vi "2D_Plotter_MATLAB.vi"(1 "Job Directory":path) -> (2 "Saved Automatically?":bool, 3 "Error String":string, 4 "Plot data file":path)   [LabVIEW 2022 SP3]
uses:
  Controls/Global_mode.ctl
  Data plotting/MATLAB/MATLAB_Mode.ctl
  <vilib>/Analysis/baseanly.llb/Mean (DBL).vi
  <vilib>/Utility/error.llb/Trim Whitespace One-Sided.vi
  Results_plotter_Global.vi
  Globals/Constants_global.vi
  Data plotting/subVIs/Plot_Values_Global.vi
  <vilib>/Analysis/NI_AALBase.lvlib
panel:
  out "Show all Axis":bool
  out "Output format":string
  out "mSingleColorbar Actual":bool=TRUE
  out "Data Filenames":path[](array[path])
  out "Ord strngs":string[](array[string])
  out "Data Dir":string[](array[string])
  out "Output file":path
  out "Duplicate Plot":bool
  out "Source locations":string[](array[string])
  out "Selectors":i32[](array[numeric])
  out "Wind Directions":dbl[](array[numeric])
  out "Max dimension per figure":dbl[](array[numeric])
  out "Max Min array":dbl[][][](array[numeric])
  out "stl Limits":sgl[][](array[numeric])
  out "All Z":dbl[](array[numeric])
  out "All Y":dbl[](array[numeric])
  out "All X":dbl[](array[numeric])
  out "C limits":dbl[][](array[numeric])
  out "Plot Titles":string[](array[string])
  out "Number of Figures":i32
  out "Plot Y Axis":i32[](array[numeric])
  out "Plot X Axis":i32[](array[numeric])
  out "Limits Array":dbl[][][](array[numeric])
  out "Constant Axis":i32[](array[numeric])
  out "Plot":i32[](array[numeric])
  out "X Labels":bool[](array[boolean])
  out "Y labels":bool[](array[boolean])
  in  "Tab Control":T1(tab)
  in  "Show Save Option?":bool
  in  "Font Size":string="10"
  in  "MainTitleFontSize":string="12"
  in  "Height":string="0.02"
  in  "Width":string="0.2"
  in  "BottomEdge":string="0.05"
  in  "LeftEdge":string="0.4"
  in  "Flip vertical and Horizontal axes":bool
  in  "Auto":bool=TRUE
  in  "Number of Contours":i8=20 min=2 max=100
  in  "Interactive Window":bool
  in  "Show Source":bool
  in  "Source Size":string="300"
  in  "Source Color":string="r"
  in  "Source Z Location":u16(ring) items=["None", "Yaw (deg)", "Pitch (deg)", "P0 (Pa)", "P1 (Pa)", "P2 (Pa)", "P3 (Pa)", "P4 (Pa)", "P5 (Pa)", "P6 (Pa)", "Pstat (Pa)", "density for calculations", "P_ref (Pa)", "ngrid desired_resolution Polynomial_fitting", "OutputFile Decimal_Places", "Uref (m/s)", "density (kg/m^3)", "User Comments", "P_atmos (mbar)", "T_external (deg C)", "T_board (deg C)", "Humidity (%)", "ax (g)", "ay (g)", "az (g)", "wx (deg / s)", "wy (deg / s)", "wz (deg / s)", "Reference Temperature Used for Corrections", "Atmos Pressure Used for Corrections", "Raw Data Filename", "Multi Run Start Time", "P0/Pref", "P1/Pref", "P2/Pref", "P3/Pref", "P4/Pref", "P5/Pref", "P6/Pref", "P0 / P0", "P1 / P0", "P2 / P0", "P3 / P0", "P4 / P0", "P5 / P0", "P6 / P0", "File", "Current Filepath", "Template File Used", "Seconds since 1st Jan", "Mano (P0) Variance p0^2", "Mano (P1) Variance p1^2", "Mano (P2) Variance p2^2", "Mano (P3) Variance p3^2", "Mano (P4) Variance p4^2", "Mano (P5) Variance p5^2", "Mano (P6) Variance p6^2", "Date", "Mano (1P0) 1P0 Zero Offset", "Mano (1P1) 1P1 Zero Offset", "Mano (1P2) 1P2 Zero Offset", "Mano (1P3) 1P3 Zero Offset", "Mano (1P4) 1P4 Zero Offset", "Mano (1P5) 1P5 Zero Offset", "Mano (1P6) 1P6 Zero Offset", "Speed Calib Tweak", "Speed Dem Voltage", "Run Description", "Multi Run Row Number", "P0 (Pa) Std Error", "P1 (Pa) Std Error", "P2 (Pa) Std Error", "P3 (Pa) Std Error", "P4 (Pa) Std Error", "P5 (Pa) Std Error", "P6 (Pa) Std Error", "P0/Pref Std Error", "P1/Pref Std Error", "P2/Pref Std Error", "P3/Pref Std Error", "P4/Pref Std Error", "P5/Pref Std Error", "P6/Pref Std Error", "Flow Measurement Time"]
  in  "Source Y Location":u16(ring) items=["None", "Yaw (deg)", "Pitch (deg)", "P0 (Pa)", "P1 (Pa)", "P2 (Pa)", "P3 (Pa)", "P4 (Pa)", "P5 (Pa)", "P6 (Pa)", "Pstat (Pa)", "density for calculations", "P_ref (Pa)", "ngrid desired_resolution Polynomial_fitting", "OutputFile Decimal_Places", "Uref (m/s)", "density (kg/m^3)", "User Comments", "P_atmos (mbar)", "T_external (deg C)", "T_board (deg C)", "Humidity (%)", "ax (g)", "ay (g)", "az (g)", "wx (deg / s)", "wy (deg / s)", "wz (deg / s)", "Reference Temperature Used for Corrections", "Atmos Pressure Used for Corrections", "Raw Data Filename", "Multi Run Start Time", "P0/Pref", "P1/Pref", "P2/Pref", "P3/Pref", "P4/Pref", "P5/Pref", "P6/Pref", "P0 / P0", "P1 / P0", "P2 / P0", "P3 / P0", "P4 / P0", "P5 / P0", "P6 / P0", "File", "Current Filepath", "Template File Used", "Seconds since 1st Jan", "Mano (P0) Variance p0^2", "Mano (P1) Variance p1^2", "Mano (P2) Variance p2^2", "Mano (P3) Variance p3^2", "Mano (P4) Variance p4^2", "Mano (P5) Variance p5^2", "Mano (P6) Variance p6^2", "Date", "Mano (1P0) 1P0 Zero Offset", "Mano (1P1) 1P1 Zero Offset", "Mano (1P2) 1P2 Zero Offset", "Mano (1P3) 1P3 Zero Offset", "Mano (1P4) 1P4 Zero Offset", "Mano (1P5) 1P5 Zero Offset", "Mano (1P6) 1P6 Zero Offset", "Speed Calib Tweak", "Speed Dem Voltage", "Run Description", "Multi Run Row Number", "P0 (Pa) Std Error", "P1 (Pa) Std Error", "P2 (Pa) Std Error", "P3 (Pa) Std Error", "P4 (Pa) Std Error", "P5 (Pa) Std Error", "P6 (Pa) Std Error", "P0/Pref Std Error", "P1/Pref Std Error", "P2/Pref Std Error", "P3/Pref Std Error", "P4/Pref Std Error", "P5/Pref Std Error", "P6/Pref Std Error", "Flow Measurement Time"]
  in  "Source X Location":u16(ring) items=["None", "Yaw (deg)", "Pitch (deg)", "P0 (Pa)", "P1 (Pa)", "P2 (Pa)", "P3 (Pa)", "P4 (Pa)", "P5 (Pa)", "P6 (Pa)", "Pstat (Pa)", "density for calculations", "P_ref (Pa)", "ngrid desired_resolution Polynomial_fitting", "OutputFile Decimal_Places", "Uref (m/s)", "density (kg/m^3)", "User Comments", "P_atmos (mbar)", "T_external (deg C)", "T_board (deg C)", "Humidity (%)", "ax (g)", "ay (g)", "az (g)", "wx (deg / s)", "wy (deg / s)", "wz (deg / s)", "Reference Temperature Used for Corrections", "Atmos Pressure Used for Corrections", "Raw Data Filename", "Multi Run Start Time", "P0/Pref", "P1/Pref", "P2/Pref", "P3/Pref", "P4/Pref", "P5/Pref", "P6/Pref", "P0 / P0", "P1 / P0", "P2 / P0", "P3 / P0", "P4 / P0", "P5 / P0", "P6 / P0", "File", "Current Filepath", "Template File Used", "Seconds since 1st Jan", "Mano (P0) Variance p0^2", "Mano (P1) Variance p1^2", "Mano (P2) Variance p2^2", "Mano (P3) Variance p3^2", "Mano (P4) Variance p4^2", "Mano (P5) Variance p5^2", "Mano (P6) Variance p6^2", "Date", "Mano (1P0) 1P0 Zero Offset", "Mano (1P1) 1P1 Zero Offset", "Mano (1P2) 1P2 Zero Offset", "Mano (1P3) 1P3 Zero Offset", "Mano (1P4) 1P4 Zero Offset", "Mano (1P5) 1P5 Zero Offset", "Mano (1P6) 1P6 Zero Offset", "Speed Calib Tweak", "Speed Dem Voltage", "Run Description", "Multi Run Row Number", "P0 (Pa) Std Error", "P1 (Pa) Std Error", "P2 (Pa) Std Error", "P3 (Pa) Std Error", "P4 (Pa) Std Error", "P5 (Pa) Std Error", "P6 (Pa) Std Error", "P0/Pref Std Error", "P1/Pref Std Error", "P2/Pref Std Error", "P3/Pref Std Error", "P4/Pref Std Error", "P5/Pref Std Error", "P6/Pref Std Error", "Flow Measurement Time"]
  in  "Rotate Model?":bool
  in  "Vectors":bool
  in  "Streamlines":bool
  in  "W Vector":u16(ring) items=["None", "Yaw (deg)", "Pitch (deg)", "P0 (Pa)", "P1 (Pa)", "P2 (Pa)", "P3 (Pa)", "P4 (Pa)", "P5 (Pa)", "P6 (Pa)", "Pstat (Pa)", "density for calculations", "P_ref (Pa)", "ngrid desired_resolution Polynomial_fitting", "OutputFile Decimal_Places", "Uref (m/s)", "density (kg/m^3)", "User Comments", "P_atmos (mbar)", "T_external (deg C)", "T_board (deg C)", "Humidity (%)", "ax (g)", "ay (g)", "az (g)", "wx (deg / s)", "wy (deg / s)", "wz (deg / s)", "Reference Temperature Used for Corrections", "Atmos Pressure Used for Corrections", "Raw Data Filename", "Multi Run Start Time", "P0/Pref", "P1/Pref", "P2/Pref", "P3/Pref", "P4/Pref", "P5/Pref", "P6/Pref", "P0 / P0", "P1 / P0", "P2 / P0", "P3 / P0", "P4 / P0", "P5 / P0", "P6 / P0", "File", "Current Filepath", "Template File Used", "Seconds since 1st Jan", "Mano (P0) Variance p0^2", "Mano (P1) Variance p1^2", "Mano (P2) Variance p2^2", "Mano (P3) Variance p3^2", "Mano (P4) Variance p4^2", "Mano (P5) Variance p5^2", "Mano (P6) Variance p6^2", "Date", "Mano (1P0) 1P0 Zero Offset", "Mano (1P1) 1P1 Zero Offset", "Mano (1P2) 1P2 Zero Offset", "Mano (1P3) 1P3 Zero Offset", "Mano (1P4) 1P4 Zero Offset", "Mano (1P5) 1P5 Zero Offset", "Mano (1P6) 1P6 Zero Offset", "Speed Calib Tweak", "Speed Dem Voltage", "Run Description", "Multi Run Row Number", "P0 (Pa) Std Error", "P1 (Pa) Std Error", "P2 (Pa) Std Error", "P3 (Pa) Std Error", "P4 (Pa) Std Error", "P5 (Pa) Std Error", "P6 (Pa) Std Error", "P0/Pref Std Error", "P1/Pref Std Error", "P2/Pref Std Error", "P3/Pref Std Error", "P4/Pref Std Error", "P5/Pref Std Error", "P6/Pref Std Error", "Flow Measurement Time"]
  in  "U Vector":u16(ring) items=["None", "Yaw (deg)", "Pitch (deg)", "P0 (Pa)", "P1 (Pa)", "P2 (Pa)", "P3 (Pa)", "P4 (Pa)", "P5 (Pa)", "P6 (Pa)", "Pstat (Pa)", "density for calculations", "P_ref (Pa)", "ngrid desired_resolution Polynomial_fitting", "OutputFile Decimal_Places", "Uref (m/s)", "density (kg/m^3)", "User Comments", "P_atmos (mbar)", "T_external (deg C)", "T_board (deg C)", "Humidity (%)", "ax (g)", "ay (g)", "az (g)", "wx (deg / s)", "wy (deg / s)", "wz (deg / s)", "Reference Temperature Used for Corrections", "Atmos Pressure Used for Corrections", "Raw Data Filename", "Multi Run Start Time", "P0/Pref", "P1/Pref", "P2/Pref", "P3/Pref", "P4/Pref", "P5/Pref", "P6/Pref", "P0 / P0", "P1 / P0", "P2 / P0", "P3 / P0", "P4 / P0", "P5 / P0", "P6 / P0", "File", "Current Filepath", "Template File Used", "Seconds since 1st Jan", "Mano (P0) Variance p0^2", "Mano (P1) Variance p1^2", "Mano (P2) Variance p2^2", "Mano (P3) Variance p3^2", "Mano (P4) Variance p4^2", "Mano (P5) Variance p5^2", "Mano (P6) Variance p6^2", "Date", "Mano (1P0) 1P0 Zero Offset", "Mano (1P1) 1P1 Zero Offset", "Mano (1P2) 1P2 Zero Offset", "Mano (1P3) 1P3 Zero Offset", "Mano (1P4) 1P4 Zero Offset", "Mano (1P5) 1P5 Zero Offset", "Mano (1P6) 1P6 Zero Offset", "Speed Calib Tweak", "Speed Dem Voltage", "Run Description", "Multi Run Row Number", "P0 (Pa) Std Error", "P1 (Pa) Std Error", "P2 (Pa) Std Error", "P3 (Pa) Std Error", "P4 (Pa) Std Error", "P5 (Pa) Std Error", "P6 (Pa) Std Error", "P0/Pref Std Error", "P1/Pref Std Error", "P2/Pref Std Error", "P3/Pref Std Error", "P4/Pref Std Error", "P5/Pref Std Error", "P6/Pref Std Error", "Flow Measurement Time"]
  in  "V Vector":u16(ring) items=["None", "Yaw (deg)", "Pitch (deg)", "P0 (Pa)", "P1 (Pa)", "P2 (Pa)", "P3 (Pa)", "P4 (Pa)", "P5 (Pa)", "P6 (Pa)", "Pstat (Pa)", "density for calculations", "P_ref (Pa)", "ngrid desired_resolution Polynomial_fitting", "OutputFile Decimal_Places", "Uref (m/s)", "density (kg/m^3)", "User Comments", "P_atmos (mbar)", "T_external (deg C)", "T_board (deg C)", "Humidity (%)", "ax (g)", "ay (g)", "az (g)", "wx (deg / s)", "wy (deg / s)", "wz (deg / s)", "Reference Temperature Used for Corrections", "Atmos Pressure Used for Corrections", "Raw Data Filename", "Multi Run Start Time", "P0/Pref", "P1/Pref", "P2/Pref", "P3/Pref", "P4/Pref", "P5/Pref", "P6/Pref", "P0 / P0", "P1 / P0", "P2 / P0", "P3 / P0", "P4 / P0", "P5 / P0", "P6 / P0", "File", "Current Filepath", "Template File Used", "Seconds since 1st Jan", "Mano (P0) Variance p0^2", "Mano (P1) Variance p1^2", "Mano (P2) Variance p2^2", "Mano (P3) Variance p3^2", "Mano (P4) Variance p4^2", "Mano (P5) Variance p5^2", "Mano (P6) Variance p6^2", "Date", "Mano (1P0) 1P0 Zero Offset", "Mano (1P1) 1P1 Zero Offset", "Mano (1P2) 1P2 Zero Offset", "Mano (1P3) 1P3 Zero Offset", "Mano (1P4) 1P4 Zero Offset", "Mano (1P5) 1P5 Zero Offset", "Mano (1P6) 1P6 Zero Offset", "Speed Calib Tweak", "Speed Dem Voltage", "Run Description", "Multi Run Row Number", "P0 (Pa) Std Error", "P1 (Pa) Std Error", "P2 (Pa) Std Error", "P3 (Pa) Std Error", "P4 (Pa) Std Error", "P5 (Pa) Std Error", "P6 (Pa) Std Error", "P0/Pref Std Error", "P1/Pref Std Error", "P2/Pref Std Error", "P3/Pref Std Error", "P4/Pref Std Error", "P5/Pref Std Error", "P6/Pref Std Error", "Flow Measurement Time"]
  in  "Stl File":u16(ring) items=["", "Case1.stl", "Case2.stl", "Case2a.stl", "Case2b.stl", "Case2c.stl", "Case3.stl", "MagicBuildingswithRoofs.stl", "StreetCanyonGeometry.stl", "Veg_Barrier_EmptyCanyon.stl", "Veg_Barrier_tree_nospacing.stl", "Veg_Barrier_tree_spacing.stl"]
  out "Y Limit":string
  out "X Limit":string
  in  "Concentration?":bool
  in  "Range Auto":bool=TRUE
  in  "Same Location limits for all plots":bool=TRUE
  in  "Swop Series and Plots":bool
  in  "mSingleColorbar":bool=TRUE
  in  "Y Limits Auto":bool=TRUE
  in  "X Limits Auto":bool=TRUE
  in  "cContourAct":bool=TRUE
  in  "Location X limits":string="-2000;2000"
  out "stl file":string
  in  "nRows":u8=3 min=1
  in  "nCols":u8=3 min=1
  in  "cScatterAct":bool=TRUE
  in  "cScatterPointSize":string="5"
  in  "Plotting":enum8{"Lin", "Log"}(ring)
  in  "fvectorRotation":string="0;0;0"
  in  "cdColorbarRange":string="0.01;100"
  in  "No Of decades":i32=3 min=1 max=10
  in  "Location Y limits":string="-2000;2000"
  in  "Open in Acrobat":bool=TRUE
  in  "Reduce Individual Plot Title Lengths if too long":bool=TRUE
  in  "Show Channels with range of Values?":bool
  in  "Page Title Pre Block":string
  in  "Page Title Post Block":string
  in  "Values to include in Page Title":i32[](listbox)
  out "Final Title":string
  in  "Math titles":bool=TRUE
  out "Plot Legends Auto":string[](array[string])
  out "No of Series supplied":i32
  out "AuditTrail":string[](array[string])
  out "Desired Legends":string[][](array[string])
  out "Table":string[][](table)
  # "Plot XY axes control"
  # "Color Bar"
  # "Overall Page Title"
  # "There are as many graphs as there are titles (from Selector 2)...."
  # "Plot Styles"
  # "Each graph contains plots from Selector 1..."
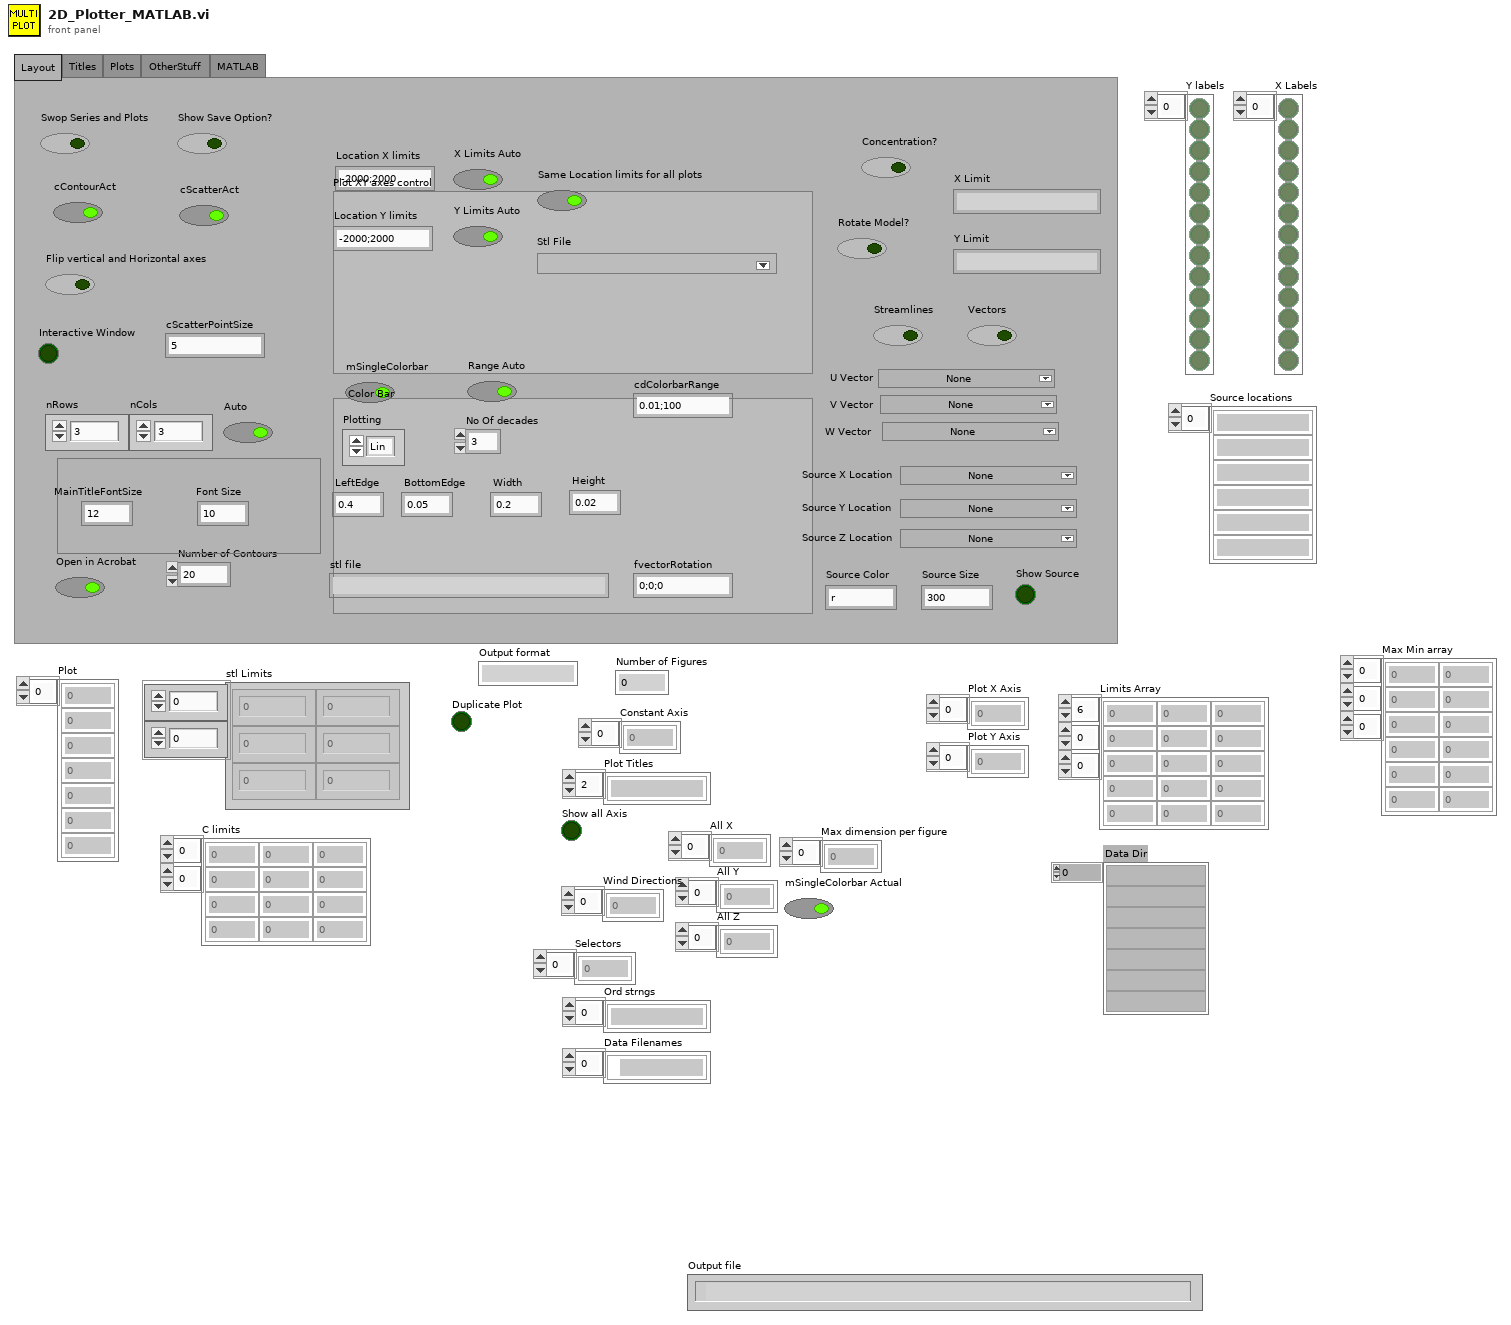
[diagram p1: front panel]
types:
  T1 = enum32{"Layout", "Titles", "Plots", "OtherStuff ", "MATLAB"}
  T2 = typedef "Global_mode.ctl" = enum16{"Read Global", "Load Global From File", "Write Global to File"}
  T3 = typedef "MATLAB_Mode.ctl" = enum16{"1D Plotter", "2D Plotter", "LP Plotter", "7HP UVW"}
  T4 = typedef "RFP_Plot_Metadata.ctl" = cluster{"Row Number":i32[], "Error Bars":T5, "X Label":string, "Y Label":string, "Blanks NaNs":i32[]}
  T5 = typedef "Error_bars_index.ctl" = cluster{"Upper":i32, "Lower":i32, "St Error":i32}
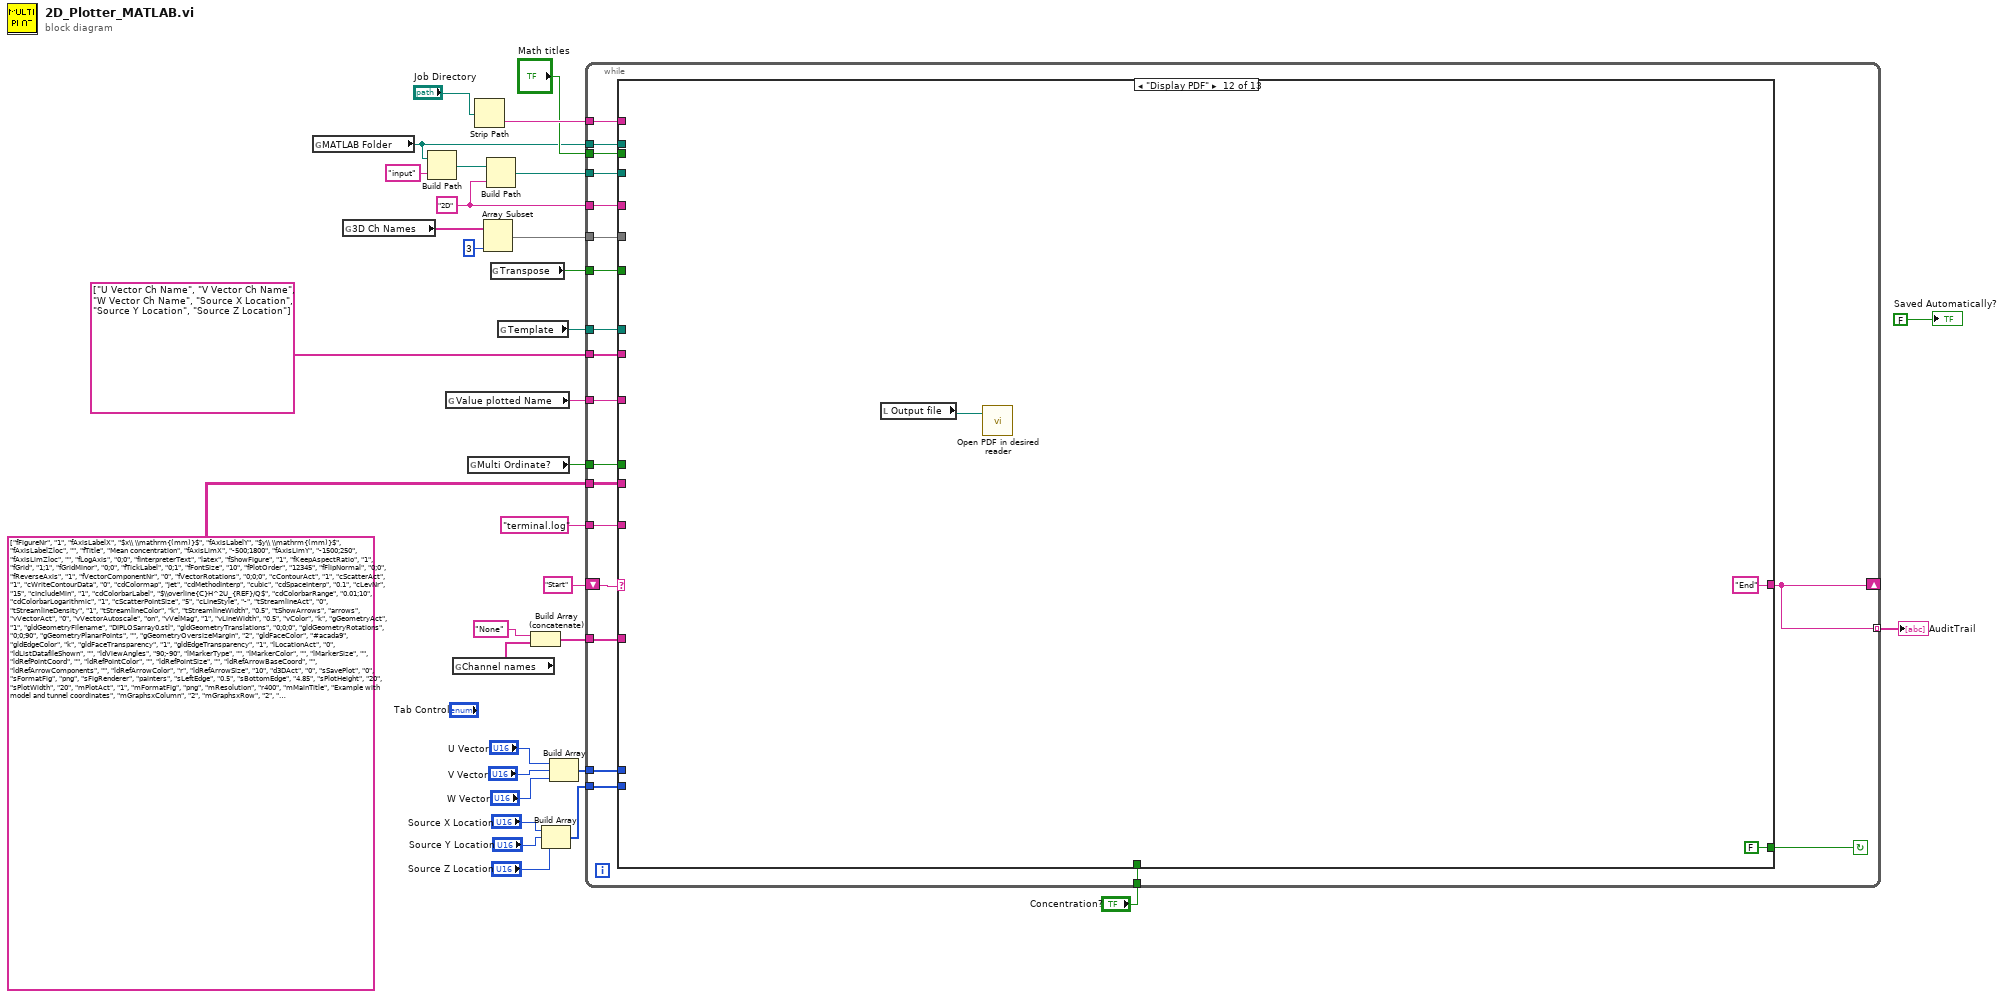
[diagram p0: block diagram]
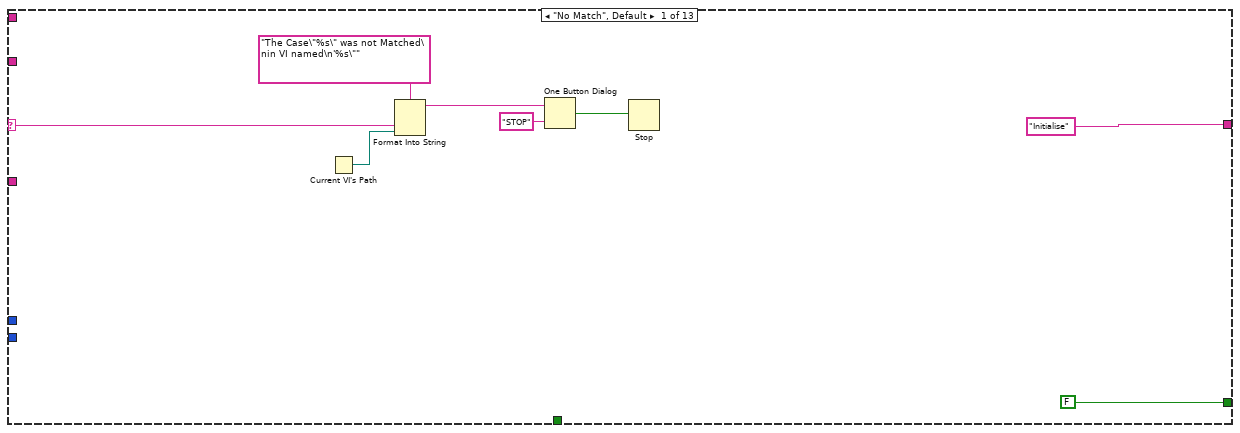
[diagram p2: hidden frame]
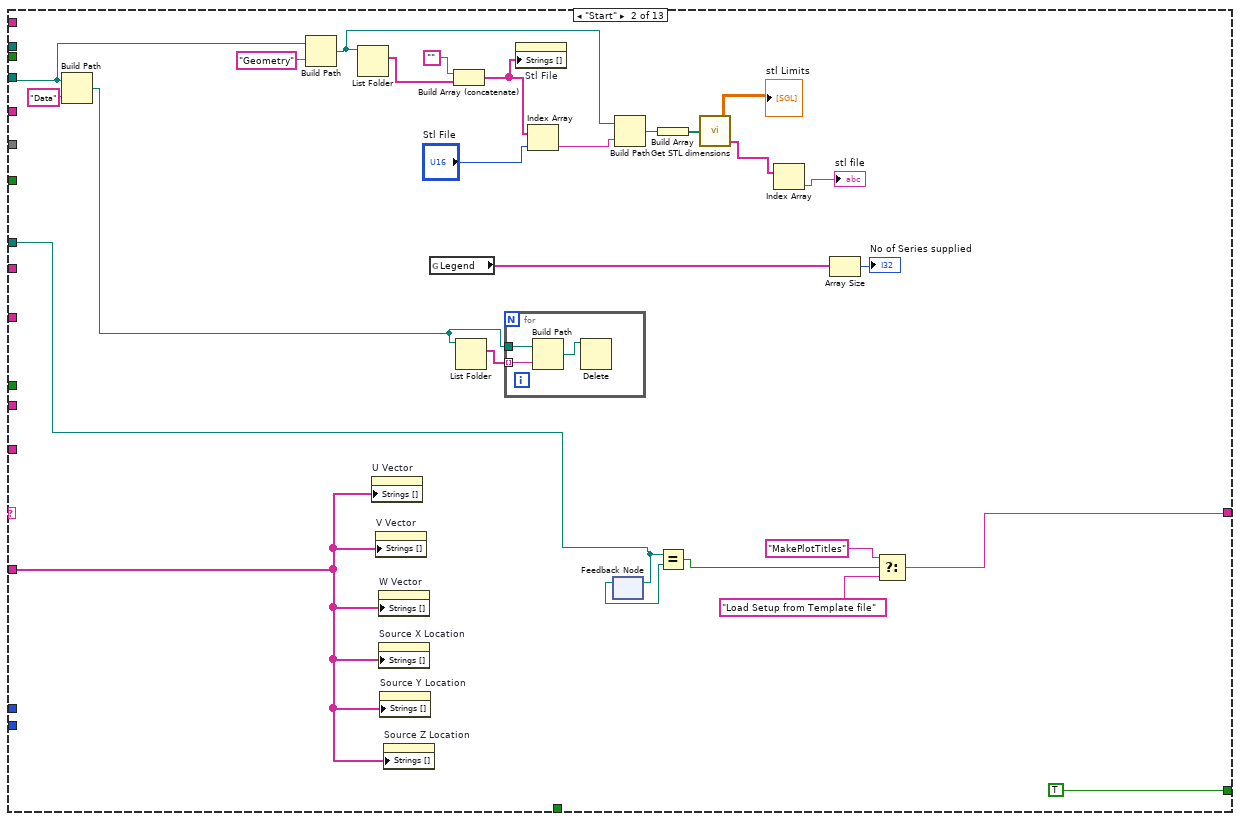
[diagram p3: hidden frame]
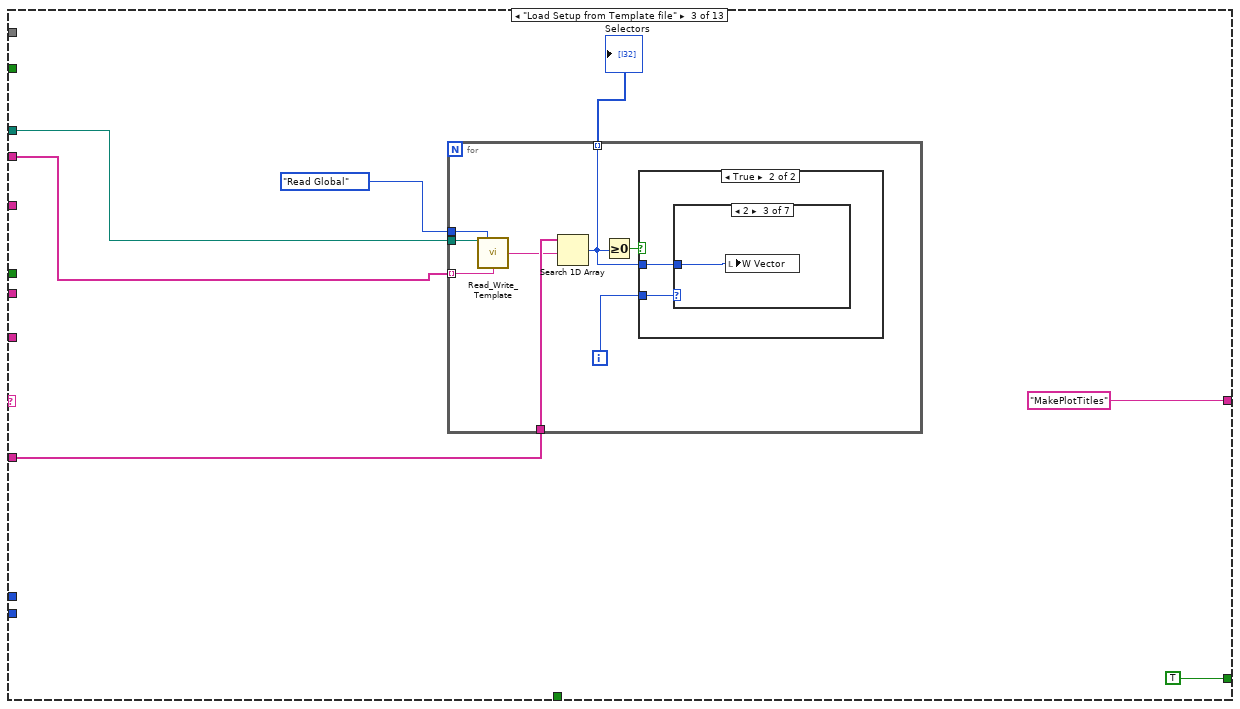
[diagram p4: hidden frame]
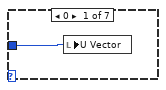
[diagram p6: hidden frame]
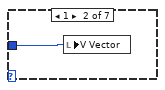
[diagram p7: hidden frame]
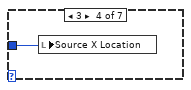
[diagram p8: hidden frame]
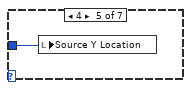
[diagram p9: hidden frame]
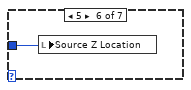
[diagram p10: hidden frame]
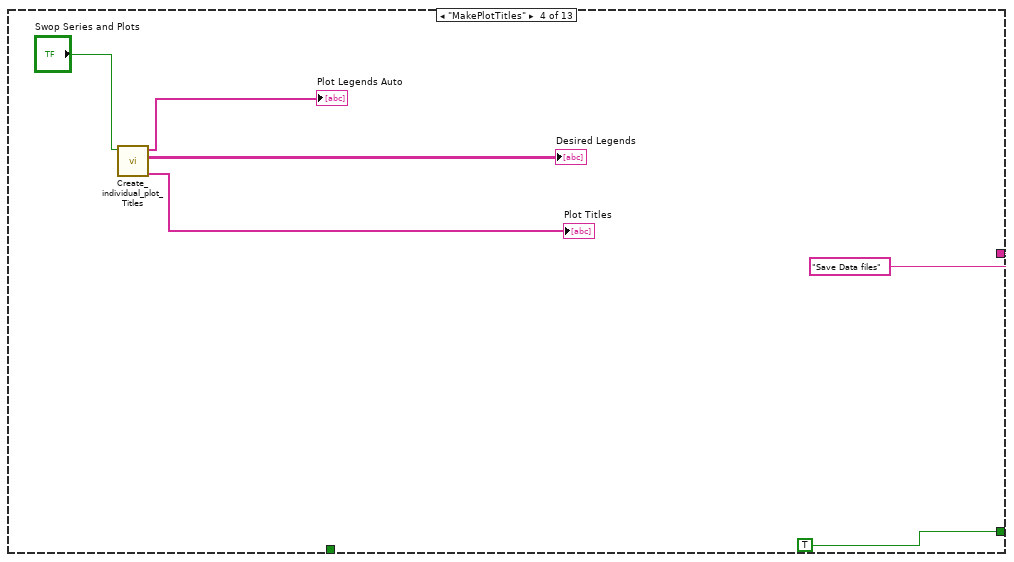
[diagram p12: hidden frame]
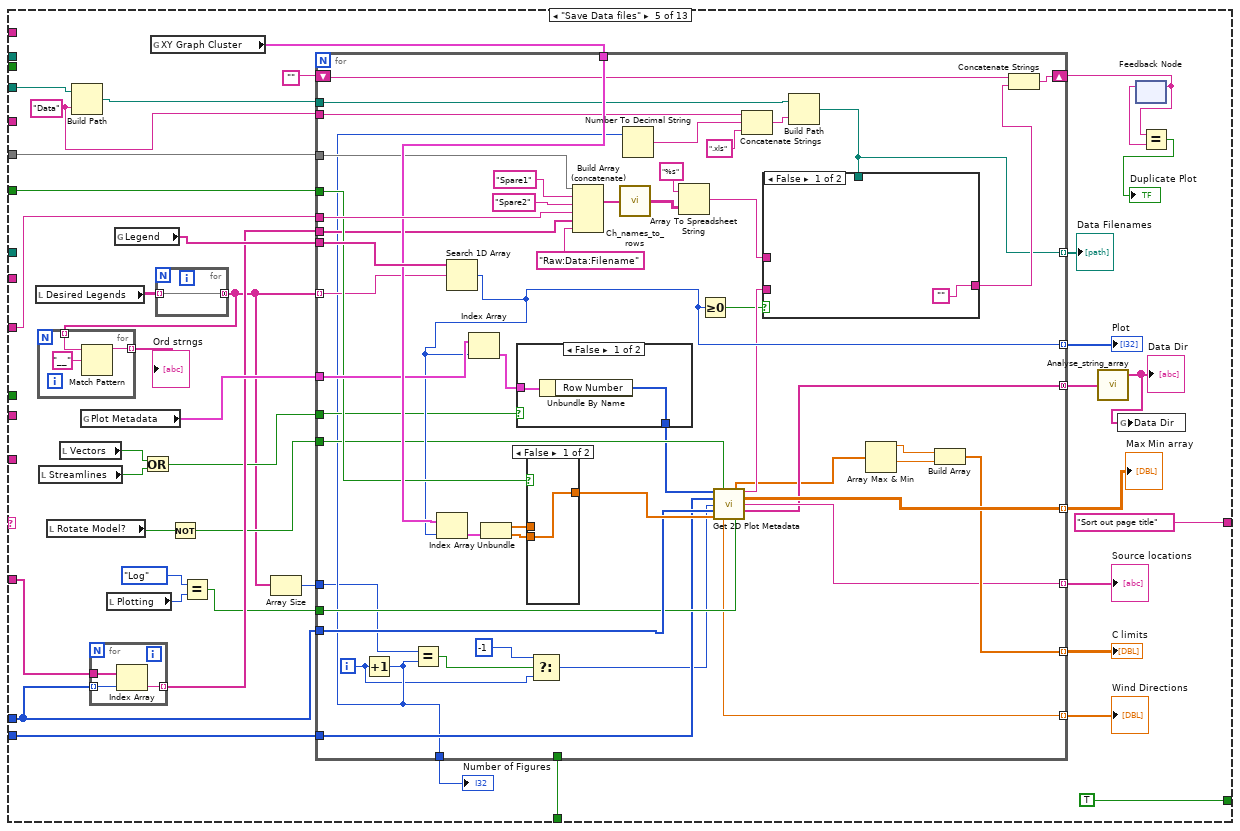
[diagram p13: hidden frame]
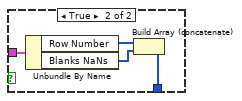
[diagram p14: hidden frame]
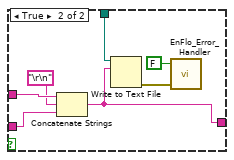
[diagram p16: hidden frame]
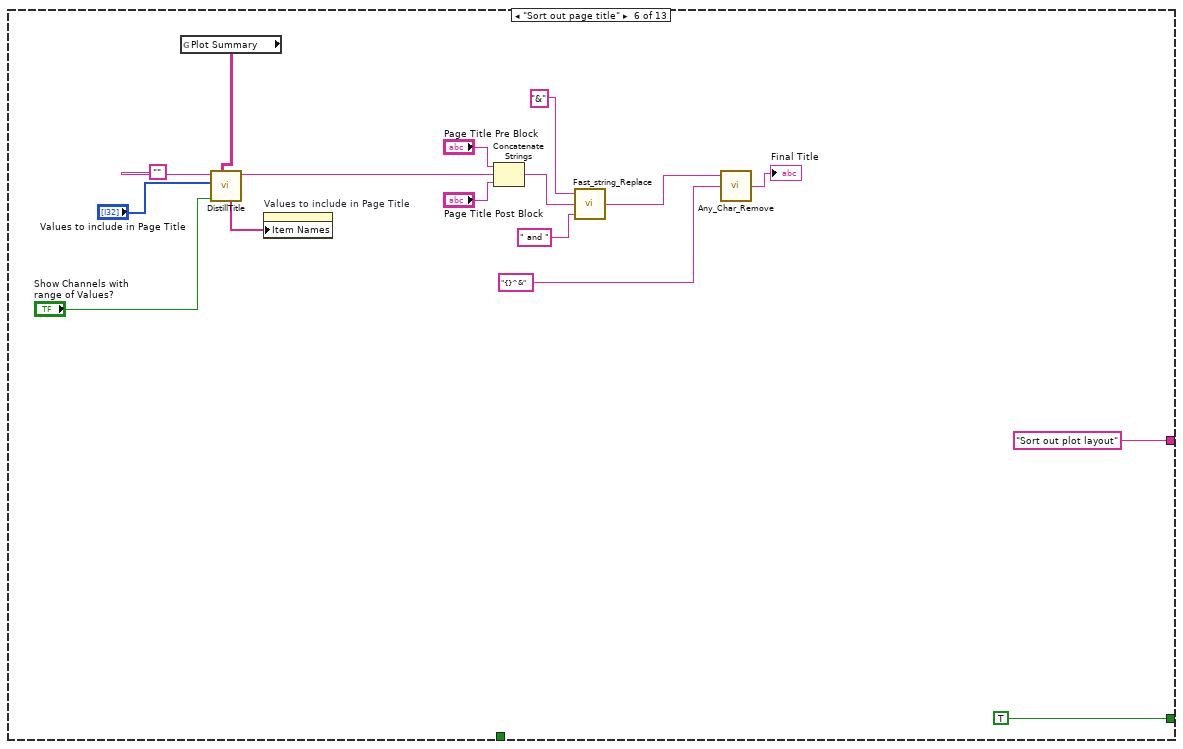
[diagram p17: hidden frame]
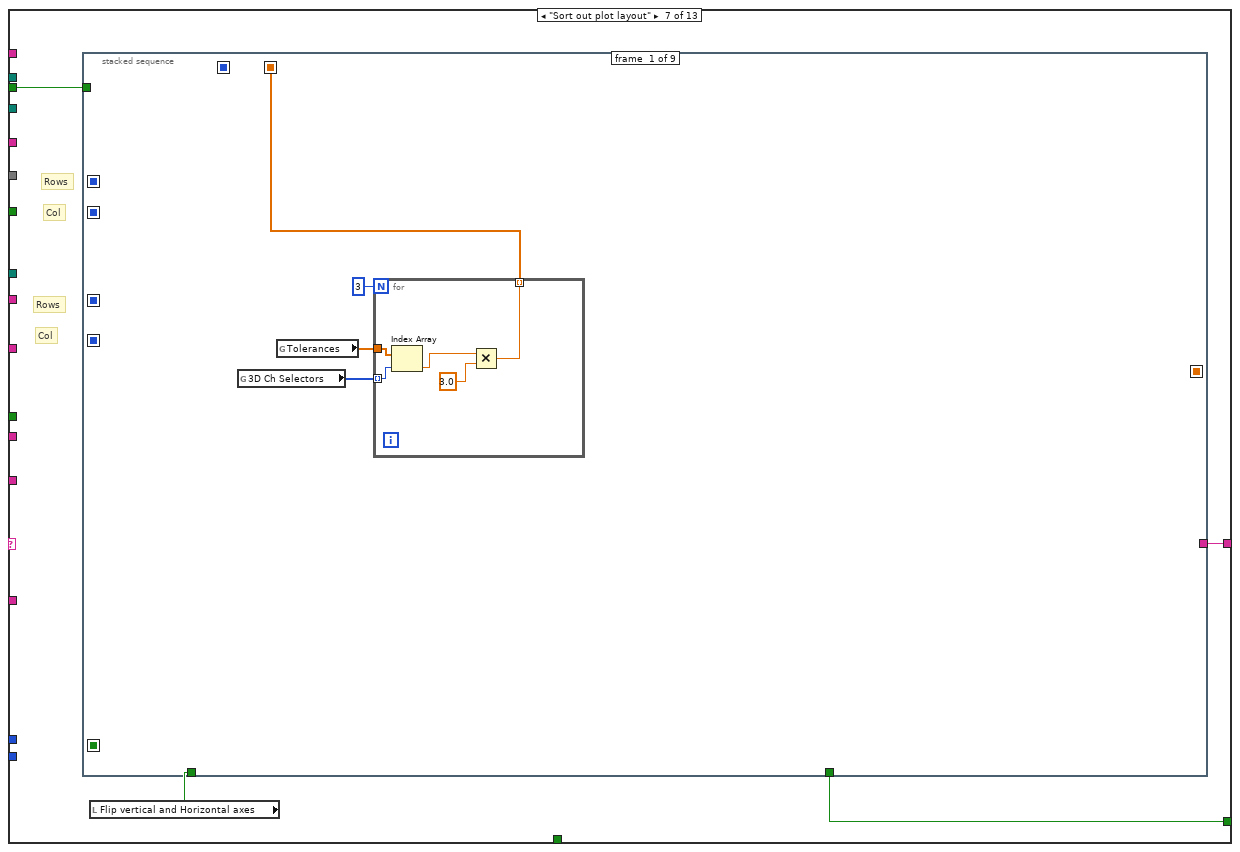
[diagram p18: hidden frame]
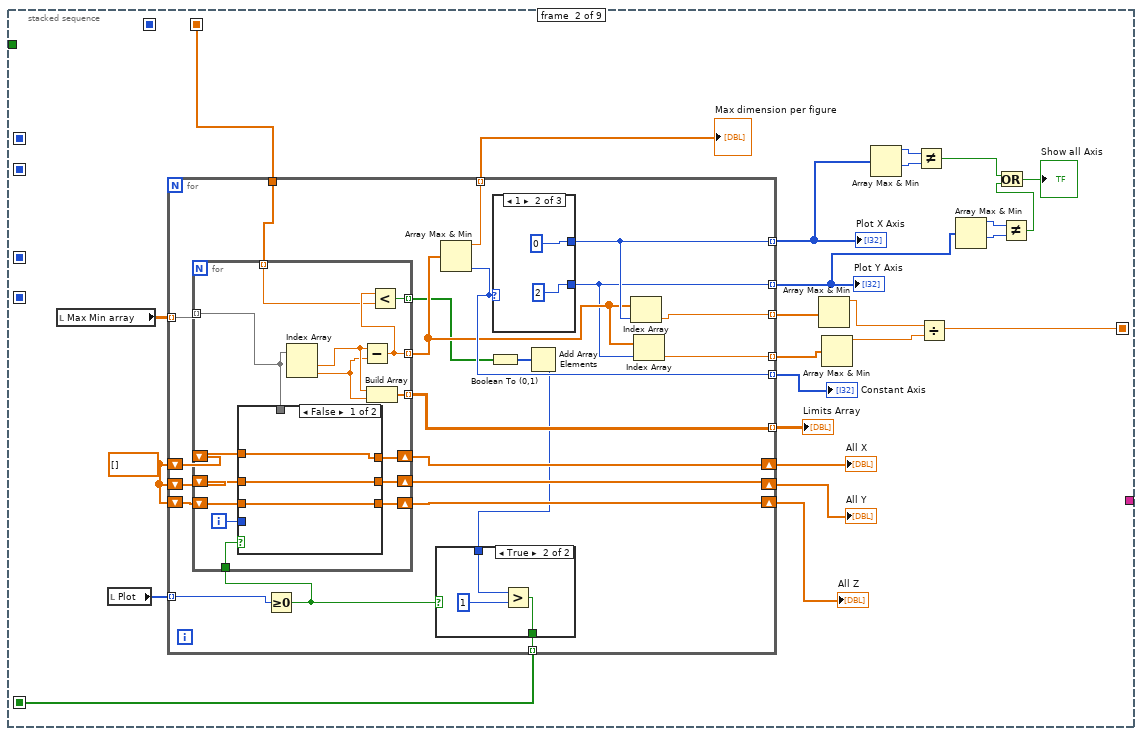
[diagram p19: hidden frame]
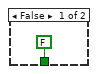
[diagram p20: hidden frame]
diagram:
  w1 = "2D" ("name or relative path")
  n1 = global read "Constants_global.vi" "MATLAB Folder"() -> (w2:path)
  n2 = global read "Results_plotter_Global.vi" "3D Ch Names"() -> (w13:string[])
  n3 = Build Path(base path=w2, name or relative path="input") -> (appended path=w25:path)
  n4 = global read "Results_plotter_Global.vi" "Value plotted Name"() -> (w32:string)
  n5 = global read "Results_plotter_Global.vi" "Channel names"() -> (w21:string[])
  n6 = global read "Results_plotter_Global.vi" "Multi Ordinate?"() -> (w28:bool)
  n7 = Strip Path(path="Job Directory") -> (name=w4:string)  [unwired: 1 out]
  n8 = Array Subset(array=w13, length=3) -> (w12:string[])  [unwired: 1 in]
  n9 = Build Path(base path=w25, name or relative path=w1) -> (appended path=w24:path)
  n10 = global read "Results_plotter_Global.vi" "Transpose"() -> (w29:bool)
  n11 = global read "Results_plotter_Global.vi" "Template"() -> (w11:path)
  n12 = Build Array (concatenate)("None", w21) -> (w19:string[])
  n13 = Build Array("Source X Location", "Source Y Location", "Source Z Location") -> (w6:u16[])
  n14 = Build Array("U Vector", "V Vector", "W Vector") -> (w15:u16[])
  n15 = while {
    shift-left: "Start" -> [w52]
    shift-right: [w47] -> _
    tunnel: w32 -> [w51]
    tunnel: "terminal.log" -> [w50]
    tunnel: w29 -> [w49]
    tunnel: w28 -> [w48]
    tunnel: [w47] -> w27 mode=indexing
    tunnel: w24 -> [w46]
    tunnel: string[][] [["fFigureNr", "1"], ["fAxisLabelX", "$x\\ \\mathrm{(mm)}$"], ["fAxisLabelY", "$y\\ \\mathrm{(mm)}$"], ["fAxisLabelZloc", ""], ["fTitle", "Mean concentration"], ["fAxisLimX", "-500;1800"], ["fAxisLimY", "-1500;250"], ["fAxisLimZloc", ""], ["fLogAxis", "0;0"], ["fInterpreterText", "latex"], ["fShowFigure", "1"], ["fKeepAspectRatio", "1"], ["fGrid", "1;1"], ["fGridMinor", "0;0"], ["fTickLabel", "0;1"], ["fFontSize", "10"], ["fPlotOrder", "12345"], ["fFlipNormal", "0;0"], ["fReverseAxis", "1"], ["fVectorComponentNr", "0"], ["fVectorRotations", "0;0;0"], ["cContourAct", "1"], ["cScatterAct", "1"], ["cWriteContourData", "0"], ["cdColormap", "jet"], ["cdMethodInterp", "cubic"], ["cdSpaceInterp", "0.1"], ["cLevNr", "15"], ["cIncludeMin", "1"], ["cdColorbarLabel", "$\\overline{C}H^2U_{REF}/Q$"], ["cdColorbarRange", "0.01;10"], ["cdColorbarLogarithmic", "1"], ["cScatterPointSize", "5"], ["cLineStyle", "-"], ["tStreamlineAct", "0"], ["tStreamlineDensity", "1"], ["tStreamlineColor", "k"], ["tStreamlineWidth", "0.5"], ["tShowArrows", "arrows"], ["vVectorAct", "0"], ["vVectorAutoscale", "on"], ["vVelMag", "1"], ["vLineWidth", "0.5"], ["vColor", "k"], ["gGeometryAct", "1"], ["gldGeometryFilename", "DIPLOSarray0.stl"], ["gldGeometryTranslations", "0;0;0"], ["gldGeometryRotations", "0;0;90"], ["gGeometryPlanarPoints", ""], ["gGeometryOversizeMargin", "2"], ["gldFaceColor", "#acada9"], ["gldEdgeColor", "k"], ["gldFaceTransparency", "1"], ["gldEdgeTransparency", "1"], ["lLocationAct", "0"], ["ldListDatafileShown", ""], ["ldViewAngles", "90;-90"], ["lMarkerType", ""], ["lMarkerColor", ""], ["lMarkerSize", ""], ["ldRefPointCoord", ""], ["ldRefPointColor", ""], ["ldRefPointSize", ""], ["ldRefArrowBaseCoord", ""], ["ldRefArrowComponents", ""], ["ldRefArrowColor", "r"], ["ldRefArrowSize", "10"], ["d3DAct", "0"], ["sSavePlot", "0"], ["sFormatFig", "png"], ["sFigRenderer", "painters"], ["sLeftEdge", "0.5"], ["sBottomEdge", "4.85"], ["sPlotHeight", "20"], ["sPlotWidth", "20"], ["mPlotAct", "1"], ["mFormatFig", "png"], ["mResolution", "r400"], ["mMainTitle", "Example with model and tunnel coordinates"], ["mGraphsxColumn", "2"], ["mGraphsxRow", "2"], ["mLeftEdge", "1.8"], ["mRightEdge", "0.8"], ["mTopEdge", "1.5"], ["mBottomEdge", "1.5"], ["mSpaceX", "0.1"], ["mSpaceY", "0.5"], ["mPlotHeight", "21"], ["mPlotWidth", "29.7"], ["mMainTitleFontSize", "12"], ["mFontSize", "10"], ["mInterpreterText", "latex"], ["mFigRenderer", "opengl"], ["mSingleColorbar", "1"], ["mSingleColorbarOrientation", "Horizontal"], ["mSingleColorbarLocation", "0.4;0.05;0.2;0.02"], ["dStreamlineSlice", "2"], ["dStreamlineStartPoint1", "0;0;0.5"], ["dStreamlineStartPoint2", "0;1;0.5"], ["dContourTransparency", "1"]] ("appended array") -> [w45]
    tunnel: "Concentration?" -> [w44]
    tunnel: w19 -> [w43]
    tunnel: w15 -> [w42]
    tunnel: w12 -> [w41]
    tunnel: w11 -> [w40]
    tunnel: string[] ["U Vector Ch Name", "V Vector Ch Name", "W Vector Ch Name", "Source X Location", "Source Y Location", "Source Z Location"] -> [w39]
    tunnel: w6 -> [w38]
    tunnel: w4 -> [w37]
    tunnel: "Math titles" -> [w36]
    tunnel: w2 -> [w35]
    tunnel: w1 -> [w34]
    stop <- w53 continue-if-true
    n16 = case shown="\"Display PDF\"" w52 {
      selector: w52 -> [w54 _ _ _ _ _ _ _ _ _ _ _ _]
      tunnel: [FALSE TRUE TRUE ("Top Level") TRUE ("Top Level") TRUE ("Top Level") TRUE ("Top Level") w255 TRUE ("Top Level") TRUE ("Top Level") w1307 FALSE ("Top Level") FALSE ("Top Level") FALSE ("Top Level")] -> w53
      tunnel: ["Initialise" w68 "MakePlotTitles" "Save Data files" "Sort out page title" "Sort out plot layout" w253 "Save Input File" ("t") "Run MATLAB Code" ("t") w1300 "" "End" ("t") "End" ("t")] -> w47
      tunnel: w51 -> [_ _ _ _ w150 _ _ _ _ _ _ _ _]
      tunnel: w50 -> [_ _ _ _ _ _ _ _ _ _ _ _ _]
      tunnel: w49 -> [_ _ _ _ w160 _ _ _ _ _ _ _ _]
      tunnel: w48 -> [_ _ _ _ _ _ _ _ _ _ _ _ _]
      tunnel: w46 -> [_ w78 _ _ w154 _ _ w792 w1280 _ _ _ _]
      tunnel: w45 -> [_ _ _ _ _ _ _ w799 _ _ _ _ _]
      tunnel: w44 -> [_ _ _ _ w147 _ _ _ _ _ _ _ _]
      tunnel: w43 -> [_ w65 w94 _ w146 _ _ _ w1268 _ _ _ _]
      tunnel: w42 -> [_ _ _ _ w144 _ _ _ _ _ _ _ _]
      tunnel: w41 -> [_ _ _ _ w143 _ _ _ _ _ _ _ _]
      tunnel: w40 -> [_ w66 w95 _ _ _ _ _ w1270 _ _ _ _]
      tunnel: w39 -> [_ _ w93 _ _ _ _ _ w1269 _ _ _ _]
      tunnel: w38 -> [_ _ _ _ w134 _ _ _ _ _ _ _ _]
      tunnel: w37 -> [_ _ _ _ _ _ _ w791 _ w1306 _ _ _]
      tunnel: w36 -> [_ _ _ _ _ _ w252 _ _ _ _ _ _]
      tunnel: w35 -> [_ _ _ _ _ _ _ _ w1260 _ _ _ _]
      tunnel: w34 -> [_ _ _ _ _ _ _ _ w1259 _ _ _ _]
      frame "No Match", Default {
        n17 = Current VI's Path() -> (path=w56:path)
        n18 = Format Into String(format string="The Case\"%s\" was not Matched\nin VI named\n'%s\"" ("Format String"), w54, w56) -> (resulting string=w59:string)  [unwired: 2 in, 1 out]
        n19 = One Button Dialog(message=w59, button name ("OK")="STOP") -> (true=w57:bool)
        n20 = Stop(stop? (T)=w57) -> ()
      }
      frame "Start" {
        n21 = Build Path(base path=w78, name or relative path="Data") -> (appended path=w82:path)
        n22 = Build Path(base path=w78, name or relative path="Geometry") -> (appended path=w73:path)
        n23 = List Folder(path=w73) -> (filenames=w79:string[])  [unwired: 3 in, 3 out]
        n24 = property on="U Vector" class="Ring (strict)"("Strings []"=w65) -> ()  [unwired: 2 in, 2 out]
        n25 = property on="V Vector" class="Ring (strict)"("Strings []"=w65) -> ()  [unwired: 2 in, 2 out]
        n26 = property on="W Vector" class="Ring (strict)"("Strings []"=w65) -> ()  [unwired: 2 in, 2 out]
        n27 = property on="Source X Location" class="Ring (strict)"("Strings []"=w65) -> ()  [unwired: 2 in, 2 out]
        n28 = property on="Source Y Location" class="Ring (strict)"("Strings []"=w65) -> ()  [unwired: 2 in, 2 out]
        n29 = property on="Source Z Location" class="Ring (strict)"("Strings []"=w65) -> ()  [unwired: 2 in, 2 out]
        n30 = global read "Results_plotter_Global.vi" "Legend"() -> (w85:string[])
        n31 = Build Array (concatenate)("", w79) -> (w71:string[])
        n32 = List Folder(path=w82) -> (filenames=w84:string[])  [unwired: 3 in, 3 out]
        n33 = for {
          tunnel: w84 -> [w90] mode=indexing
          tunnel: w82 -> [w89]
          n34 = Build Path(base path=w89, name or relative path=w90) -> (appended path=w88:path)
          n35 = Delete(path (use dialog)=w88) -> ()  [unwired: 4 in, 3 out]
        }
        n36 = property on="Stl File" class="Ring (strict)"("Strings []"=w71) -> ()  [unwired: 2 in, 2 out]
        n37 = Index Array(array=w71, index="Stl File") -> (element=w72:string)
        n38 = feedback #1() -> (w67:path)  [unwired: 1 in]
        n39 = feedback-in #1(w66) -> ()
        n40 = Build Path(base path=w73, name or relative path=w72) -> (appended path=w74:path)
        n41 = Build Array(w74) -> (w76:path[])
        n42 = Equal?(x=w66, y=w67) -> (x = y?=w70:bool)
        n43 = call "Get STL dimensions.vi"("Stl Filenames"=w76) -> ("Limits"=→"stl Limits":sgl[][], "stl Files"=w64:string[])  [unwired: 1 out]
        n44 = Index Array(array=w64) -> (element=→"stl file":string)  [unwired: 1 in]
        n45 = Array Size(array=w85) -> (size(s)=→"No of Series supplied":i32)
        n46 = Select(t="MakePlotTitles", s=w70, f="Load Setup from Template file") -> (s? t:f=w68:string)
      }
      frame "Load Setup from Template file" {
        n47 = for {
          tunnel: w95 -> [w105]
          tunnel: Global_mode."Read Global" ("Mode") -> [w104]
          tunnel: w93 -> [w103] mode=indexing
          tunnel: w94 -> [w102]
          tunnel: [w98] -> w97 mode=indexing
          i -> [w100]
          n48 = call "Read_Write_Template.vi"("Template File"=w105, "Mode"=w104, "Data type"=w103) -> ("Single Value Out"=w101:string)  [unwired: 5 in, 7 out]
          n49 = Search 1D Array(1D array=w102, element=w101) -> (index of element=w98:i32)  [unwired: 1 in]
          n50 = Greater Or Equal To 0?(x=w98) -> (x >= 0?=w99:bool)
          n51 = case shown="True" w99 {
            tunnel: w100 -> [_ w107]
            tunnel: w98 -> [_ w106]
            frame False {
            }
            frame True {
              n52 = case shown="2" w107 {
                tunnel: w106 -> [w108 w109 w110 w111 w112 w113 _]
                frame 0 {
                  n53 = local write "U Vector"(w108) -> ()
                }
                frame 1 {
                  n54 = local write "V Vector"(w109) -> ()
                }
                frame 2 {
                  n55 = local write "W Vector"(w110) -> ()
                }
                frame 3 {
                  n56 = local write "Source X Location"(w111) -> ()
                }
                frame 4 {
                  n57 = local write "Source Y Location"(w112) -> ()
                }
                frame 5 {
                  n58 = local write "Source Z Location"(w113) -> ()
                }
                frame Default {
                }
              }
            }
          }
        }
        "Selectors" <- w97
      }
      frame "MakePlotTitles" {
        n59 = call "Create_individual_plot_Titles.vi"("Swop Series and Plots"="Swop Series and Plots") -> ("2D Plot Titles"=→"Plot Titles":string[], "Desired Legends"=→"Desired Legends":string[][], "Plot Legends Auto"=→"Plot Legends Auto":string[])  [unwired: 2 in, 2 out]
      }
      frame "Save Data files" {
        w153 = "Data" ("name or relative path")
        n60 = local read "Desired Legends"() -> (w149:string[][])
        n61 = local read "Streamlines"() -> (w127:bool)
        n62 = local read "Rotate Model?"() -> (w137:bool)
        n63 = local read "Vectors"() -> (w126:bool)
        n64 = Build Path(base path=w154, name or relative path=w153) -> (appended path=w152:path)
        n65 = global read "Results_plotter_Global.vi" "Plot Metadata"() -> (w155:T4[])
        n66 = for {
          tunnel: w144 -> [w166] mode=indexing
          tunnel: w146 -> [w165]
          tunnel: [w164] -> w145 mode=indexing
          n67 = Index Array(array=w165, index=w166) -> (element=w164:string)
        }
        n68 = local read "Plotting"() -> (w141:enum8{"Lin", "Log"})
        n69 = global read "Results_plotter_Global.vi" "Legend"() -> (w156:string[])
        n70 = Or(x=w126, y=w127) -> (x .or. y?=w125:bool)
        n71 = global read "Plot_Values_Global.vi" "XY Graph Cluster"() -> (w135:cluster{dbl[], dbl[]}[])
        n72 = for {
          tunnel: w149 -> [w167] mode=indexing
          tunnel: [w167] -> w121 mode=concatenating
        }
        n73 = for {
          tunnel: w121 -> [w163] mode=indexing
          tunnel: [w161] -> w124 mode=indexing
          n74 = Match Pattern(string=w163, regular expression="__") -> (before substring=w161:string)  [unwired: 1 in, 3 out]
        }
        "Ord strngs" <- w124
        n75 = Not(x=w137) -> (.not. x?=w136:bool)
        n76 = Equal?(x=enum8{"Lin", "Log"}."Log" ("Plotting"), y=w141) -> (x = y?=w140:bool)
        n77 = Array Size(array=w121) -> (size(s)=w120:i32)
        n78 = for {
          tunnel: w160 -> [w202]
          tunnel: w135 -> [w212]
          tunnel: [w173] -> w157
          tunnel: w150 -> [w217]
          tunnel: w156 -> [w213]
          tunnel: w121 -> [w199] mode=indexing
          tunnel: w155 -> [w210]
          tunnel: w153 -> [w205]
          tunnel: w152 -> [w203]
          tunnel: [w198] -> w151 mode=indexing
          tunnel: [w185] -> w148 mode=indexing
          tunnel: w147 -> [_]
          tunnel: w145 -> [w196]
          tunnel: w144 -> [w193]
          tunnel: w143 -> [w195]
          tunnel: w140 -> [w192]
          tunnel: [w190] -> w139 mode=indexing
          tunnel: [w189] -> w138 mode=indexing
          tunnel: w136 -> [w188]
          tunnel: w134 -> [w184]
          tunnel: [w183] -> w133 mode=indexing
          shift-right: [w181] -> w130
          shift-left: "" -> [w182]
          tunnel: [w180] -> w128 mode=concatenating
          tunnel: w125 -> [w176]
          tunnel: [w174] -> w123 mode=indexing
          tunnel: w120 -> [w172]
          i -> [w170]
          n79 = Increment(x=w170) -> (x+1=w173:i32)
          n80 = Equal?(x=w172, y=w173) -> (x = y?=w171:bool)
          n81 = Search 1D Array(1D array=w213, element=w199) -> (index of element=w198:i32)  [unwired: 1 in]
          n82 = Index Array(array=w212, index=w198) -> (element=w211:cluster{dbl[], dbl[]})
          n83 = Index Array(array=w210, index=w198) -> (element=w209:T4)
          n84 = Unbundle(w211) -> (w201:dbl[], w200:dbl[])
          n85 = case shown="False" w176 {
            tunnel: w209 -> [w221 w225]
            tunnel: [w220 w222] -> w177
            frame False {
              n86 = Unbundle By Name(w221) -> ("Row Number"=w220:i32[])
            }
            frame True {
              n87 = Unbundle By Name(w225) -> ("Row Number"=w224:i32[], "Blanks NaNs"=w223:i32[])
              n88 = Build Array (concatenate)(w224, w223) -> (w222:i32[])
            }
          }
          n89 = case shown="False" w202 {
            tunnel: [w226 w227] -> w194
            tunnel: w201 -> [_ w227]
            tunnel: w200 -> [w226 _]
            frame False {
            }
            frame True {
            }
          }
          n90 = Select(t=-1, s=w171, f=w170) -> (s? t:f=w169:i32)
          n91 = Build Array (concatenate)(w195, "Spare1", "Spare2", w217, w196, "Raw:Data:Filename" ("element")) -> (w214:string[])
          n92 = call "Ch_names_to_rows.vi"("Channel Names"=w214) -> ("3 Row names"=w216:string[][])
          n93 = Number To Decimal String(number=w173) -> (decimal integer string=w206:string)  [unwired: 1 in]
          n94 = Array To Spreadsheet String(array=w216, 3:"%s" ("format string")) -> (spreadsheet string=w208:string)  [unwired: 1 out]
          n95 = Greater Or Equal To 0?(x=w198) -> (x >= 0?=w175:bool)
          n96 = call "Get 2D Plot Metadata.vi"("Row Number"=w177, "Model?"=w188, "Source Location"=w184, "Interation number"=w169, "UVW index"=w193, "Scalar Value"=w194, "Log Plot?"=w192) -> ("Scalar limits"=w179:dbl[], "spreadsheet string"=w191:string, "Max Min array"=w190:dbl[][], "Source Location"=w183:string, "Data Directories"=w180:string[], "Wind Direction"=w189:dbl)  [unwired: 2 in, 1 out]
          n97 = Concatenate Strings(w205, w206, ".xls" ("string")) -> (w204:string)
          n98 = Build Path(base path=w203, name or relative path=w204) -> (appended path=w174:path)
          n99 = case shown="False" w175 {
            tunnel: w208 -> [_ w235]
            tunnel: w191 -> [_ w234]
            tunnel: ["" w232] -> w178
            tunnel: w174 -> [_ w229]
            frame False {
            }
            frame True {
              n100 = Concatenate Strings(w235, "\r\n", w234) -> (w232:string)
              n101 = Write to Text File(file (use dialog)=w229, text=w232) -> (error out=w231:errorcluster)  [unwired: 2 in, 2 out]
              n102 = call "EnFlo_Error_Handler.vi"("error in (no error)"=w231, "Dialog Box (F)"=FALSE ("Dialog Box (T)")) -> ()  [unwired: 2 in, 2 out]
            }
          }
          n103 = Array Max & Min(array=w179) -> (max value=w187:dbl, min value=w186:dbl)  [unwired: 2 out]
          n104 = Build Array(w187, w186) -> (w185:dbl[])
          n105 = Concatenate Strings(w182, w178) -> (w181:string)
        }
        "Number of Figures" <- w157
        "Plot" <- w151
        "C limits" <- w148
        "Max Min array" <- w139
        "Wind Directions" <- w138
        "Source locations" <- w133
        "Data Filenames" <- w123
        n106 = call "Analyse_string_array.vi"("String array"=w128) -> ("Unique strings"=w122:string[])  [unwired: 1 in, 1 out]
        "Data Dir" <- w122
        n107 = global write "Results_plotter_Global.vi" "Data Dir"(w122) -> ()
        n108 = feedback #2() -> (w131:string)  [unwired: 1 in]
        n109 = feedback-in #2(w130) -> ()
        n110 = Equal?(x=w130, y=w131) -> (x = y?=→"Duplicate Plot":bool)
      }
      frame "Sort out page title" {
        n111 = global read "Results_plotter_Global.vi" "Plot Summary"() -> (w237:string[][])
        n112 = call "DistillTitle.vi"("Plot Summary in"=w237, "Show Channels with range of Values?"="Show Channels with range of Values?", "Indices to include in Page Title"="Values to include in Page Title", "String in"="") -> ("String out"=w250:string, "AvailableVariables"=w245:string[])  [unwired: 6 in]
        n113 = property on="Values to include in Page Title" class="LstBox (strict)"("Item Names"=w245) -> ()  [unwired: 2 in, 2 out]
        n114 = Concatenate Strings("Page Title Pre Block", w250, "Page Title Post Block") -> (w241:string)
        n115 = call "Fast_string_Replace.vi"("Replace match with:"=" and " ("Individual Characters to Remove"), "Input String"=w241, "matchThis"="&" ("Individual Characters to Remove")) -> ("Output String"=w238:string)  [unwired: 1 in, 1 out]
        n116 = call "Any_Char_Remove.vi"("Individual Characters to Remove"="{}^&", "String in"=w238) -> ("String out"=→"Final Title":string)  [unwired: 1 in]
      }
      frame "Sort out plot layout" {
        # "Col"
        # "Rows"
        # "Col"
        # "Rows"
        n117 = local read "Flip vertical and Horizontal axes"() -> (w254:bool)
        n118 = stacked-sequence {
          seq-local: [_ _ w365 _ _ _ _ _ _] -> [_ _ _ w373 _ _ _ _ _]
          seq-local: [_ _ w364 _ _ _ _ _ _] -> [_ _ _ w371 _ _ _ _ _]
          seq-local: [_ _ _ w374 _ _ _ _ _] -> [_ _ _ _ w665 _ _ _ _]
          seq-local: [_ _ _ w372 _ _ _ _ _] -> [_ _ _ _ w664 _ w717 _ _]
          seq-local: [_ _ w363 _ _ _ _ _ _] -> [_ _ _ w370 w663 _ _ _ _]
          seq-local: [_ w283 _ _ _ _ _ _ _] -> [_ _ _ _ _ w709 _ _ _]
          seq-local: [_ w276 _ _ _ _ _ _ _] -> [_ _ _ w368 _ _ _ _ _]
          seq-local: [w256 _ _ _ _ _ _ _ _] -> [_ w275 _ _ _ _ _ _ _]
          tunnel: [_ _ _ _ _ w707 _ _ _] -> w255
          tunnel: w254 -> [_ _ _ w366 w672 _ _ _ _]
          tunnel: [_ _ _ _ "Create Input file" _ _ _ _] -> w253
          tunnel: w252 -> [_ _ _ _ _ _ w713 _ _]
          frame #0 {
            n119 = global read "Results_plotter_Global.vi" "3D Ch Selectors"() -> (w257:i32[])
            n120 = global read "Results_plotter_Global.vi" "Tolerances"() -> (w258:dbl[])
            n121 = for {
              N: 3 -> [_]
              tunnel: w258 -> [w264]
              tunnel: w257 -> [w263] mode=indexing
              tunnel: [w260] -> w256 mode=indexing
              n122 = Index Array(array=w264, index=w263) -> (element=w262:dbl)
              n123 = Multiply(x=w262, y=3.0) -> (x*y=w260:dbl)
            }
          }
          frame #1 {
            w287 = dbl[] []
            n124 = local read "Max Min array"() -> (w282:dbl[][][])
            n125 = local read "Plot"() -> (w274:i32[])
            n126 = for {
              tunnel: [w304] -> w289 mode=indexing
              tunnel: [w311] -> w288 mode=indexing
              tunnel: [w298] -> w271 mode=indexing
              tunnel: [w296] -> w268 mode=indexing
              shift-right: [w309] -> w286
              shift-left: w287 -> [w310]
              shift-right: [w306] -> w285
              shift-left: w287 -> [w308]
              shift-right: [w305] -> w284
              shift-left: w287 -> [w307]
              tunnel: [w301] -> w283 mode=indexing
              tunnel: w282 -> [w300] mode=indexing
              tunnel: [w299] -> w281 mode=indexing
              tunnel: [w295] -> w280 mode=indexing
              tunnel: [w294] -> w279 mode=indexing
              tunnel: w275 -> [w293]
              tunnel: w274 -> [w291] mode=indexing
              n127 = Greater Or Equal To 0?(x=w291) -> (x >= 0?=w290:bool)
              n128 = for {
                tunnel: [w325] -> w297 mode=indexing
                tunnel: [w335] -> w311 mode=indexing
                shift-right: [w332] -> w309
                shift-left: w310 -> [w333]
                shift-right: [w331] -> w306
                shift-left: w308 -> [w330]
                shift-right: [w329] -> w305
                shift-left: w307 -> [w328]
                tunnel: w300 -> [w327] mode=indexing
                tunnel: w293 -> [w324] mode=indexing
                tunnel: [w323] -> w292 mode=indexing
                tunnel: w290 -> [w322]
                i -> [w334]
                n129 = case shown="False" w322 {
                  tunnel: w334 -> [_ w347]
                  tunnel: w333 -> [w339 w346]
                  tunnel: [w339 w345] -> w332
                  tunnel: [w338 w344] -> w331
                  tunnel: w330 -> [w338 w343]
                  tunnel: [w337 w342] -> w329
                  tunnel: w328 -> [w337 w341]
                  tunnel: w327 -> [_ w340]
                  frame False {
                  }
                  frame True {
                    n130 = case shown="1" w347 {
                      tunnel: w346 -> [w352 w357 w362]
                      tunnel: w340 -> [w351 w355 w360]
                      tunnel: [w350 w357 w362] -> w345
                      tunnel: [w349 w354 w358] -> w344
                      tunnel: w343 -> [w349 w356 w358]
                      tunnel: [w348 w353 w359] -> w342
                      tunnel: w341 -> [w348 w353 w361]
                      frame 0, Default {
                        n131 = Build Array (concatenate)(w352, w351) -> (w350:dbl[])
                      }
                      frame 1 {
                        n132 = Build Array (concatenate)(w356, w355) -> (w354:dbl[])
                      }
                      frame 2 {
                        n133 = Build Array (concatenate)(w361, w360) -> (w359:dbl[])
                      }
                    }
                  }
                }
                n134 = Index Array(array=w327) -> (element #1=w336:dbl, element #2=w326:dbl)  [unwired: 2 in]
                n135 = Subtract(x=w336, y=w326) -> (x-y=w325:dbl)
                n136 = Build Array(w336, w326) -> (w335:dbl[])
                n137 = Less?(x=w325, y=w324) -> (x < y?=w323:bool)
              }
              n138 = Array Max & Min(array=w297) -> (max value=w299:dbl, min index (indices)=w304:i32)  [unwired: 2 out]
              n139 = Boolean To (0,1)(Boolean=w292) -> (0, 1=w303:i16[])
              n140 = case shown="1" w304 {
                tunnel: [1 ("index") 0 ("index") 0 ("index")] -> w298
                tunnel: [2 ("index") 2 ("index") 1 ("index")] -> w296
                frame 0, Default {
                }
                frame 1 {
                }
                frame 2 {
                }
              }
              n141 = Add Array Elements(numeric array=w303) -> (sum=w302:i16)
              n142 = case shown="True" w290 {
                tunnel: w302 -> [_ w315]
                tunnel: [FALSE w313] -> w301
                frame False {
                }
                frame True {
                  n143 = Greater?(x=w315, y=i16 1) -> (0:w313:bool)
                }
              }
              n144 = Index Array(array=w297, index=w298) -> (element=w295:dbl)
              n145 = Index Array(array=w297, index=w296) -> (element=w294:dbl)
            }
            "Constant Axis" <- w289
            "Limits Array" <- w288
            "Plot X Axis" <- w271
            "Plot Y Axis" <- w268
            "All X" <- w286
            "All Y" <- w285
            "All Z" <- w284
            "Max dimension per figure" <- w281
            n146 = Array Max & Min(array=w280) -> (max value=w278:dbl)  [unwired: 3 out]
            n147 = Array Max & Min(array=w279) -> (max value=w277:dbl)  [unwired: 3 out]
            n148 = Array Max & Min(array=w271) -> (max value=w273:i32, min value=w272:i32)  [unwired: 2 out]
            n149 = Not Equal?(x=w273, y=w272) -> (x != y?=w266:bool)
            n150 = Divide(x=w278, y=w277) -> (x/y=w276:dbl)
            n151 = Array Max & Min(array=w268) -> (max value=w269:i32, min value=w270:i32)  [unwired: 2 out]
            n152 = Not Equal?(x=w269, y=w270) -> (x != y?=w267:bool)
            n153 = Or(x=w266, y=w267) -> (x .or. y?=→"Show all Axis":bool)
          }
          frame #2 {
            n154 = local read "Number of Figures"() -> (w363:i32)
            n155 = local read "nCols"() -> (w364:u8)
            n156 = local read "nRows"() -> (w365:u8)
          }
          frame #3 {
            n157 = case shown="True" w366 {
              tunnel: [w375 w376] -> w367
              tunnel: w368 -> [w375 w377]
              frame False {
              }
              frame True {
                n158 = Reciprocal(x=w377) -> (1/x=w376:dbl)
              }
            }
            n159 = case shown="True" "Auto" {
              tunnel: w370 -> [_ w381]
              tunnel: [w379 w383] -> w374
              tunnel: w373 -> [w379 _]
              tunnel: [w378 w382] -> w372
              tunnel: w371 -> [w378 _]
              tunnel: w367 -> [_ w380]
              frame False {
              }
              frame True {
                n160 = case shown="9" w381 {
                  tunnel: [u8 1 ("nRows") w390 w400 w417 w434 w458 w482 w506 w530 w547 w571 w595 w619 w636 w649 u8 5 ("nRows") u8 6 ("nRows")] -> w382
                  tunnel: [u8 1 ("nRows") w389 w399 w416 w433 w457 w481 w505 w529 w546 w570 w594 w618 w635 w648 u8 5 ("nRows") u8 5 ("nRows")] -> w383
                  tunnel: w380 -> [_ w388 w396 w413 w430 w454 w478 w502 w526 w543 w567 w591 w615 w632 w650 _ _]
                  frame 1 {
                  }
                  frame 2 {
                    n161 = Greater?(x=w388, y=1.9) -> (0:w386:bool)
                    n162 = case shown="True" w386 {
                      tunnel: [u8 2 ("nRows") u8 1 ("nRows")] -> w390
                      tunnel: [u8 1 ("nRows") u8 2 ("nRows")] -> w389
                      frame False {
                      }
                      frame True {
                      }
                    }
                  }
                  frame 3 {
                    w395 = 3.0 ("upper limit")
                    n163 = In Range and Coerce(upper limit=w395, x=w396, lower limit=1.2) -> (In Range?=w397:bool)  [unwired: 1 out]
                    n164 = case shown="False" w397 {
                      tunnel: [w401 u8 2 ("nRows")] -> w400
                      tunnel: [w402 u8 2 ("nRows")] -> w399
                      tunnel: w396 -> [w405 _]
                      tunnel: w395 -> [w404 _]
                      frame False {
                        n165 = Greater?(x=w405, y=w404) -> (0:w403:bool)
                        n166 = case shown="False" w403 {
                          tunnel: [u8 3 ("nRows") u8 1 ("nRows")] -> w402
                          tunnel: [u8 1 ("nRows") u8 3 ("nRows")] -> w401
                          frame True {
                          }
                          frame False {
                          }
                        }
                      }
                      frame True {
                      }
                    }
                  }
                  frame 4 {
                    w412 = 4.5 ("upper limit")
                    n167 = In Range and Coerce(upper limit=w412, x=w413, lower limit=0.89) -> (In Range?=w414:bool)  [unwired: 1 out]
                    n168 = case shown="False" w414 {
                      tunnel: [w418 u8 2 ("nRows")] -> w417
                      tunnel: [w419 u8 2 ("nRows")] -> w416
                      tunnel: w413 -> [w422 _]
                      tunnel: w412 -> [w421 _]
                      frame False {
                        n169 = Greater?(x=w422, y=w421) -> (0:w420:bool)
                        n170 = case shown="False" w420 {
                          tunnel: [u8 4 ("nRows") u8 1 ("nRows")] -> w419
                          tunnel: [u8 1 ("nRows") u8 4 ("nRows")] -> w418
                          frame True {
                          }
                          frame False {
                          }
                        }
                      }
                      frame True {
                      }
                    }
                  }
                  frame 5 {
                    w429 = 6.7 ("upper limit")
                    n171 = In Range and Coerce(upper limit=w429, x=w430, lower limit=0.73) -> (In Range?=w431:bool)  [unwired: 1 out]
                    n172 = case shown="True" w431 {
                      tunnel: [w435 w448] -> w434
                      tunnel: [w436 w447] -> w433
                      tunnel: w430 -> [w439 w446]
                      tunnel: w429 -> [w438 _]
                      frame False {
                        n173 = Greater?(x=w439, y=w438) -> (0:w437:bool)
                        n174 = case shown="True" w437 {
                          tunnel: [u8 5 ("nRows") u8 1 ("nRows")] -> w436
                          tunnel: [u8 1 ("nRows") u8 5 ("nRows")] -> w435
                          frame True {
                          }
                          frame False {
                          }
                        }
                      }
                      frame True {
                        n175 = Greater?(x=w446, y=2.5) -> (0:w444:bool)
                        n176 = case shown="False" w444 {
                          tunnel: [u8 2 ("nRows") u8 3 ("nRows")] -> w448
                          tunnel: [u8 3 ("nRows") u8 2 ("nRows")] -> w447
                          frame True {
                          }
                          frame False {
                          }
                        }
                      }
                    }
                  }
                  frame 6 {
                    w453 = 8.2 ("upper limit")
                    n177 = In Range and Coerce(upper limit=w453, x=w454, lower limit=0.59) -> (In Range?=w455:bool)  [unwired: 1 out]
                    n178 = case shown="True" w455 {
                      tunnel: [w459 w472] -> w458
                      tunnel: [w460 w471] -> w457
                      tunnel: w454 -> [w463 w470]
                      tunnel: w453 -> [w462 _]
                      frame False {
                        n179 = Greater?(x=w463, y=w462) -> (0:w461:bool)
                        n180 = case shown="False" w461 {
                          tunnel: [u8 6 ("nRows") u8 1 ("nRows")] -> w460
                          tunnel: [u8 1 ("nRows") u8 6 ("nRows")] -> w459
                          frame True {
                          }
                          frame False {
                          }
                        }
                      }
                      frame True {
                        n181 = Greater?(x=w470, y=2.5) -> (0:w468:bool)
                        n182 = case shown="False" w468 {
                          tunnel: [u8 2 ("nRows") u8 3 ("nRows")] -> w472
                          tunnel: [u8 3 ("nRows") u8 2 ("nRows")] -> w471
                          frame True {
                          }
                          frame False {
                          }
                        }
                      }
                    }
                  }
                  frame 7 {
                    w477 = 11.0 ("upper limit")
                    n183 = In Range and Coerce(upper limit=w477, x=w478, lower limit=0.5) -> (In Range?=w479:bool)  [unwired: 1 out]
                    n184 = case shown="True" w479 {
                      tunnel: [w483 w496] -> w482
                      tunnel: [w484 w495] -> w481
                      tunnel: w478 -> [w487 w494]
                      tunnel: w477 -> [w486 _]
                      frame False {
                        n185 = Greater?(x=w487, y=w486) -> (0:w485:bool)
                        n186 = case shown="True" w485 {
                          tunnel: [u8 7 ("nRows") u8 1 ("nRows")] -> w484
                          tunnel: [u8 1 ("nRows") u8 7 ("nRows")] -> w483
                          frame True {
                          }
                          frame False {
                          }
                        }
                      }
                      frame True {
                        n187 = Greater?(x=w494, y=2.5) -> (0:w492:bool)
                        n188 = case shown="True" w492 {
                          tunnel: [u8 2 ("nRows") u8 4 ("nRows")] -> w496
                          tunnel: [u8 4 ("nRows") u8 2 ("nRows")] -> w495
                          frame True {
                          }
                          frame False {
                          }
                        }
                      }
                    }
                  }
                  frame 8 {
                    w501 = 14.0 ("upper limit")
                    n189 = In Range and Coerce(upper limit=w501, x=w502, lower limit=0.45) -> (In Range?=w503:bool)  [unwired: 1 out]
                    n190 = case shown="True" w503 {
                      tunnel: [w507 w520] -> w506
                      tunnel: [w508 w519] -> w505
                      tunnel: w502 -> [w511 w518]
                      tunnel: w501 -> [w510 _]
                      frame False {
                        n191 = Greater?(x=w511, y=w510) -> (0:w509:bool)
                        n192 = case shown="False" w509 {
                          tunnel: [u8 8 ("nRows") u8 1 ("nRows")] -> w508
                          tunnel: [u8 1 ("nRows") u8 8 ("nRows")] -> w507
                          frame True {
                          }
                          frame False {
                          }
                        }
                      }
                      frame True {
                        n193 = Greater?(x=w518, y=2.1) -> (0:w516:bool)
                        n194 = case shown="True" w516 {
                          tunnel: [u8 2 ("nRows") u8 4 ("nRows")] -> w520
                          tunnel: [u8 4 ("nRows") u8 2 ("nRows")] -> w519
                          frame True {
                          }
                          frame False {
                          }
                        }
                      }
                    }
                  }
                  frame 9 {
                    w525 = 1.5 ("upper limit")
                    n195 = In Range and Coerce(upper limit=w525, x=w526, lower limit=0.7) -> (In Range?=w527:bool)  [unwired: 1 out]
                    n196 = case shown="False" w527 {
                      tunnel: [w531 u8 3 ("nRows")] -> w530
                      tunnel: [w532 u8 3 ("nRows")] -> w529
                      tunnel: w526 -> [w535 _]
                      tunnel: w525 -> [w534 _]
                      frame False {
                        n197 = Greater?(x=w535, y=w534) -> (0:w533:bool)
                        n198 = case shown="False" w533 {
                          tunnel: [u8 5 ("nRows") u8 2 ("nRows")] -> w532
                          tunnel: [u8 2 ("nRows") u8 5 ("nRows")] -> w531
                          frame True {
                          }
                          frame False {
                          }
                        }
                      }
                      frame True {
                      }
                    }
                  }
                  frame 10 {
                    w542 = 3.9 ("upper limit")
                    n199 = In Range and Coerce(upper limit=w542, x=w543, lower limit=1.12) -> (In Range?=w544:bool)  [unwired: 1 out]
                    n200 = case shown="False" w544 {
                      tunnel: [w548 w561] -> w547
                      tunnel: [w549 w560] -> w546
                      tunnel: w543 -> [w552 w559]
                      tunnel: w542 -> [w551 _]
                      frame False {
                        n201 = Greater?(x=w552, y=w551) -> (0:w550:bool)
                        n202 = case shown="False" w550 {
                          tunnel: [u8 5 ("nRows") u8 2 ("nRows")] -> w549
                          tunnel: [u8 2 ("nRows") u8 5 ("nRows")] -> w548
                          frame True {
                          }
                          frame False {
                          }
                        }
                      }
                      frame True {
                        n203 = Greater?(x=w559, y=2.1) -> (0:w557:bool)
                        n204 = case shown="False" w557 {
                          tunnel: [u8 3 ("nRows") u8 4 ("nRows")] -> w561
                          tunnel: [u8 4 ("nRows") u8 3 ("nRows")] -> w560
                          frame True {
                          }
                          frame False {
                          }
                        }
                      }
                    }
                  }
                  frame 11 {
                    w566 = 4.1 ("upper limit")
                    n205 = In Range and Coerce(upper limit=w566, x=w567, lower limit=0.94) -> (In Range?=w568:bool)  [unwired: 1 out]
                    n206 = case shown="True" w568 {
                      tunnel: [w572 w585] -> w571
                      tunnel: [w573 w584] -> w570
                      tunnel: w567 -> [w576 w583]
                      tunnel: w566 -> [w575 _]
                      frame False {
                        n207 = Greater?(x=w576, y=w575) -> (0:w574:bool)
                        n208 = case shown="True" w574 {
                          tunnel: [u8 6 ("nRows") u8 2 ("nRows")] -> w573
                          tunnel: [u8 2 ("nRows") u8 6 ("nRows")] -> w572
                          frame True {
                          }
                          frame False {
                          }
                        }
                      }
                      frame True {
                        n209 = Greater?(x=w583, y=2.1) -> (0:w581:bool)
                        n210 = case shown="False" w581 {
                          tunnel: [u8 3 ("nRows") u8 4 ("nRows")] -> w585
                          tunnel: [u8 4 ("nRows") u8 3 ("nRows")] -> w584
                          frame True {
                          }
                          frame False {
                          }
                        }
                      }
                    }
                  }
                  frame 12 {
                    w590 = 5.6 ("upper limit")
                    n211 = In Range and Coerce(upper limit=w590, x=w591, lower limit=0.94) -> (In Range?=w592:bool)  [unwired: 1 out]
                    n212 = case shown="False" w592 {
                      tunnel: [w596 w609] -> w595
                      tunnel: [w597 w608] -> w594
                      tunnel: w591 -> [w600 w607]
                      tunnel: w590 -> [w599 _]
                      frame False {
                        n213 = Greater?(x=w600, y=w599) -> (0:w598:bool)
                        n214 = case shown="False" w598 {
                          tunnel: [u8 6 ("nRows") u8 2 ("nRows")] -> w597
                          tunnel: [u8 2 ("nRows") u8 6 ("nRows")] -> w596
                          frame True {
                          }
                          frame False {
                          }
                        }
                      }
                      frame True {
                        n215 = Greater?(x=w607, y=2.1) -> (0:w605:bool)
                        n216 = case shown="False" w605 {
                          tunnel: [u8 3 ("nRows") u8 4 ("nRows")] -> w609
                          tunnel: [u8 4 ("nRows") u8 3 ("nRows")] -> w608
                          frame True {
                          }
                          frame False {
                          }
                        }
                      }
                    }
                  }
                  frame 13, 14 {
                    w614 = 5.3 ("upper limit")
                    n217 = In Range and Coerce(upper limit=w614, x=w615, lower limit=1.15) -> (In Range?=w616:bool)  [unwired: 1 out]
                    n218 = case shown="False" w616 {
                      tunnel: [w620 u8 4 ("nRows")] -> w619
                      tunnel: [w621 u8 4 ("nRows")] -> w618
                      tunnel: w615 -> [w624 _]
                      tunnel: w614 -> [w623 _]
                      frame False {
                        n219 = Greater?(x=w624, y=w623) -> (0:w622:bool)
                        n220 = case shown="True" w622 {
                          tunnel: [u8 7 ("nRows") u8 2 ("nRows")] -> w621
                          tunnel: [u8 2 ("nRows") u8 7 ("nRows")] -> w620
                          frame True {
                          }
                          frame False {
                          }
                        }
                      }
                      frame True {
                      }
                    }
                  }
                  frame 15, 16 {
                    w631 = 7.5 ("upper limit")
                    n221 = In Range and Coerce(upper limit=w631, x=w632, lower limit=0.98) -> (In Range?=w633:bool)  [unwired: 1 out]
                    n222 = case shown="True" w633 {
                      tunnel: [w637 u8 4 ("nRows")] -> w636
                      tunnel: [w638 u8 4 ("nRows")] -> w635
                      tunnel: w632 -> [w641 _]
                      tunnel: w631 -> [w640 _]
                      frame False {
                        n223 = Greater?(x=w641, y=w640) -> (0:w639:bool)
                        n224 = case shown="False" w639 {
                          tunnel: [u8 8 ("nRows") u8 2 ("nRows")] -> w638
                          tunnel: [u8 2 ("nRows") u8 8 ("nRows")] -> w637
                          frame True {
                          }
                          frame False {
                          }
                        }
                      }
                      frame True {
                      }
                    }
                  }
                  frame 17..20 {
                    n225 = Greater?(x=w650, y=1.9) -> (0:w651:bool)
                    n226 = case shown="True" w651 {
                      tunnel: [u8 5 ("nRows") u8 4 ("nRows")] -> w649
                      tunnel: [u8 4 ("nRows") u8 5 ("nRows")] -> w648
                      frame False {
                      }
                      frame True {
                      }
                    }
                  }
                  frame 21..25 {
                  }
                  frame 26, Default {
                  }
                }
              }
            }
          }
          frame #4 {
            n227 = local write "nRows"(w665) -> ()
            n228 = local write "nCols"(w664) -> ()
            n229 = for {
              N: w665 -> [_]
              tunnel: w664 -> [w693]
              tunnel: w663 -> [w692]
              tunnel: [w691] -> w666 mode=indexing
              tunnel: [w689] -> w662 mode=concatenating
              i -> [w694]
              n230 = Multiply(x=w693, y=w694) -> (x*y=w690:i32)
              n231 = for {
                N: w693 -> [_]
                tunnel: w690 -> [w702]
                tunnel: w692 -> [w701]
                tunnel: [w695] -> w691 mode=indexing
                tunnel: [w699] -> w689 mode=indexing
                i -> [w700]
                n232 = Add(x=w702, y=w700) -> (x+y=w697:i32)
                n233 = Equal To 0?(x=w700) -> (x = 0?=w699:bool)
                n234 = Less?(x=w697, y=w701) -> (x < y?=w698:bool)
                n235 = Select(t=w697, s=w698, f=-1) -> (s? t:f=w695:i32)
              }
            }
            n236 = Decrement(x=w665) -> (x-1=w667:u8)
            n237 = for {
              N: w664 -> [_]
              tunnel: w666 -> [w679]
              tunnel: w667 -> [w681]
              tunnel: [w678] -> w668 mode=indexing
              i -> [w682]
              n238 = Index Array(array=w679, index (row)=w681, index (col)=w682) -> (element=w677:i32)
              n239 = Decrement(x=w681) -> (x-1=w680:u8)
              n240 = Less Than 0?(x=w677) -> (x < 0?=w683:bool)
              n241 = case shown="False" w683 {
                tunnel: w682 -> [_ w688]
                tunnel: w680 -> [_ w687]
                tunnel: w679 -> [_ w686]
                tunnel: [w684 w685] -> w678
                tunnel: w677 -> [w684 _]
                frame False {
                }
                frame True {
                  n242 = Index Array(array=w686, index (row)=w687, index (col)=w688) -> (element=w685:i32)
                }
              }
            }
            n243 = for {
              N: w663 -> [_]
              tunnel: w668 -> [w676]
              tunnel: [w673] -> w661 mode=indexing
              i -> [w675]
              n244 = Search 1D Array(1D array=w676, element=w675) -> (index of element=w674:i32)  [unwired: 1 in]
              n245 = Greater Or Equal To 0?(x=w674) -> (x >= 0?=w673:bool)
            }
            n246 = case shown="False" w672 {
              tunnel: [w704 w705] -> w671
              tunnel: w661 -> [w704 w706]
              tunnel: [w703 w706] -> w670
              tunnel: w662 -> [w703 w705]
              frame False {
              }
              frame True {
              }
            }
            "Y labels" <- w670
            "X Labels" <- w671
          }
          frame #5 {
            n247 = Or Array Elements(Boolean array=w709) -> (logical OR=w708:bool)
            n248 = case shown="True" w708 {
              tunnel: [TRUE ("Top Level") FALSE ("Top Level")] -> w707
              frame False {
              }
              frame True {
                n249 = One Button Dialog(message="Please select plains for the 2D plotter") -> ()  [unwired: 1 in, 1 out]
              }
            }
          }
          frame #6 {
            n250 = case shown="False" w713 {
              tunnel: [140 100] -> w718
              frame False {
              }
              frame True {
              }
            }
            n251 = Divide(x=w718, y=w717) -> (x/y=w716:dbl)
            n252 = local read "Plot Titles"() -> (w715:string[])
            n253 = call "Reduce Title length.vi"("Reduce Individual Plot Title Lengths if too long"="Reduce Individual Plot Title Lengths if too long", "Array in"=w715, "No of Charcters"=w716) -> ("Array out"=w714:string[])  [unwired: 2 in]
            n254 = local write "Plot Titles"(w714) -> ()
          }
          frame #7 {
            n255 = local read "Plot"() -> (w724:i32[])
            n256 = Greater Or Equal To 0?(x=w724) -> (x >= 0?=w722:bool[])
            n257 = And Array Elements(Boolean array=w722) -> (logical AND=w723:bool)
            n258 = case shown="False" w723 {
              tunnel: w722 -> [w727 _]
              frame False {
                n259 = local read "Data Filenames"() -> (w725:path[])
                n260 = for {
                  tunnel: w727 -> [w756] mode=indexing
                  tunnel: [w755] -> w740
                  i -> [w755]
                  stop <- w756 stop-if-true
                }
                n261 = Index Array(array=w725, index=w740) -> (element=w739:path)
                n262 = Read from Text File(file (use dialog)=w739) -> (text=w738:string)  [unwired: 3 in, 3 out]
                n263 = Spreadsheet String To Array(format string="%s", spreadsheet string=w738, array type (2D Dbl)=string[][] []) -> (array=w734:string[][])  [unwired: 1 in]
                n264 = Array Subset(array=w734, index (row)=4 ("length")) -> (w732:string[][])  [unwired: 3 in]
                n265 = for {
                  tunnel: w732 -> [w748] mode=indexing
                  tunnel: [w746] -> w731 mode=indexing
                  n266 = in-place {
                    n267 = in-place-split #3(w748, 3) -> (w750:string[], w751:string[])
                    n268 = Fract/Exp String To Number(string=w750) -> (number=w754:dbl[])  [unwired: 3 in, 1 out]
                    n269 = Add(x=w754, y=1000000.0) -> (x+y=w752:dbl[])
                    n270 = Number To Fractional String(number=w752) -> (F-format string=w749:string[])  [unwired: 3 in]
                    n271 = in-place-split #3(w749, w751) -> (w746:string[])  [unwired: 1 out]
                  }
                }
                n272 = Array Subset(array=w734, length (row)=4 ("length")) -> (w730:string[][])  [unwired: 3 in]
                n273 = Build Array (concatenate)(w730, w731) -> (w729:string[][])
                n274 = Array To Spreadsheet String(array=w729, 3:"%s" ("format string")) -> (spreadsheet string=w726:string)  [unwired: 1 in]
                n275 = for {
                  tunnel: w727 -> [w743] mode=indexing
                  tunnel: w726 -> [w742]
                  tunnel: w725 -> [w741] mode=indexing
                  n276 = case shown="False" w743 {
                    tunnel: w742 -> [w745 _]
                    tunnel: w741 -> [w744 _]
                    frame False {
                      n277 = Write to Text File(file (use dialog)=w744, text=w745) -> ()  [unwired: 2 in, 3 out]
                    }
                    frame True {
                    }
                  }
                }
              }
              frame True {
              }
            }
          }
          frame #8 {
            n278 = case shown="True" "mSingleColorbar" {
              selector: "mSingleColorbar" -> [w763 _]
              tunnel: [w763 w764] -> w758
              frame False {
              }
              frame True {
                n279 = global read "Results_plotter_Global.vi" "Ordinate Strings"() -> (w768:string[])
                n280 = Array Size(array=w768) -> (size(s)=w767:i32)
                n281 = Equal?(x=w767, y=1) -> (x = y?=w765:bool)
                n282 = case shown="False" w765 {
                  tunnel: [w774 TRUE] -> w764
                  frame False {
                    n283 = local read "C limits"() -> (w784:dbl[][])
                    n284 = for {
                      tunnel: w784 -> [w789] mode=indexing
                      tunnel: [w786] -> w773 mode=indexing
                      tunnel: [w785] -> w780 mode=indexing
                      n285 = Index Array(array=w789) -> (element #1=w785:dbl, element #2=w788:dbl)  [unwired: 2 in]
                      n286 = Subtract(x=w785, y=w788) -> (x-y=w787:dbl)
                      n287 = Absolute Value(x=w787) -> (abs(x)=w786:dbl)
                    }
                    n288 = call-poly <vilib>:"Mean.vi"("X"=w773) -> ("mean"=w771:dbl)  [unwired: 1 out]
                    n289 = Array Max & Min(array=w780) -> (max value=w779:dbl, min value=w778:dbl)  [unwired: 2 out]
                    n290 = Array Max & Min(array=w773) -> (max value=w783:dbl, min value=w782:dbl)  [unwired: 2 out]
                    n291 = Subtract(x=w779, y=w778) -> (x-y=w772:dbl)
                    n292 = Divide(x=w772, y=w771) -> (x/y=w770:dbl)
                    n293 = Divide(x=w783, y=w782) -> (x/y=w777:dbl)
                    n294 = Less?(x=w770, y=0.75) -> (x < y?=w775:bool)
                    n295 = Less?(x=w777, y=3.0) -> (x < y?=w776:bool)
                    n296 = And(x=w776, y=w775) -> (x .and. y?=w774:bool)
                  }
                  frame True {
                  }
                }
              }
            }
            n297 = local read "Range Auto"() -> (w759:bool)
            n298 = case shown="False" w759 {
              tunnel: [TRUE w762] -> w757
              tunnel: w758 -> [_ w762]
              frame False {
              }
              frame True {
              }
            }
            "mSingleColorbar Actual" <- w757
          }
        }
      }
      frame "Create Input file" {
        n299 = local read "Plot"() -> (w796:i32[])
        n300 = Index Array(array=w799, index (col)=1 ("disabled index (col)")) -> (element=w797:string[])  [unwired: 1 in]
        n301 = Index Array(array=w799, index (col)=0 ("disabled index (col)")) -> (element=w794:string[])  [unwired: 1 in]
        n302 = for {
          tunnel: [w805] -> w795 mode=indexing
          tunnel: w794 -> [w810]
          tunnel: w797 -> [w809]
          tunnel: w796 -> [w807] mode=indexing
          tunnel: w792 -> [w806]
          shift-right: [w805] -> _
          shift-left: _ -> [w804]
          tunnel: w791 -> [w803]
          i -> [w808]
          n303 = for {
            tunnel: w810 -> [w819] mode=indexing
            tunnel: [w818] -> w805 mode=indexing
            tunnel: w809 -> [w817] mode=indexing
            tunnel: w808 -> [w816]
            tunnel: w807 -> [w815]
            tunnel: w806 -> [w814]
            tunnel: w804 -> [w813]
            tunnel: w803 -> [w811]
            i -> [w812]
            n304 = case shown="\"fAxisLabelY\"" w819 {
              tunnel: [w820 w831 w849 w855 w936 w942 w955 w957 w960 w964 w987 w1010 w1016 w1075 w1106 w1109 w1121 w1128 w1135 w1157 w1168 "fvectorRotation" w1176 w1177 w1180 w1188 w1192 w1199 w1203 w1206 w1210 w1212 w1214 "MainTitleFontSize" "Font Size" w1219 w1222 w1228 w1237 w1245 w1249 w1253 w1256] -> w818
              tunnel: w817 -> [_ _ _ _ _ _ _ _ _ _ _ _ _ _ _ _ _ _ _ _ _ _ _ _ _ _ _ _ _ _ _ _ _ _ _ _ _ _ _ _ _ _ w1256]
              tunnel: w816 -> [_ w829 _ w858 _ w943 _ _ _ _ w974 w997 w1020 w1076 w1107 w1111 w1123 _ w1134 w1161 _ _ _ _ w1178 _ w1196 _ _ _ _ _ _ _ _ _ _ _ _ _ _ _ _]
              tunnel: w815 -> [_ w825 _ _ _ w941 _ _ _ _ _ _ w1019 w1074 _ _ _ _ _ _ _ _ _ _ _ _ _ _ _ _ _ _ _ _ _ _ _ _ _ _ _ _ _]
              tunnel: w814 -> [_ _ _ _ _ _ _ _ _ _ _ _ _ _ _ _ _ _ _ _ _ _ _ _ _ _ _ _ _ _ _ _ _ _ _ _ _ _ _ _ _ _ _]
              tunnel: w813 -> [_ _ _ _ _ w940 _ _ _ _ _ _ w1018 w1072 _ _ _ _ _ _ _ _ _ _ _ _ _ _ _ _ _ _ _ _ _ _ _ _ _ _ _ _ _]
              tunnel: w812 -> [_ _ _ _ _ w939 _ _ _ _ _ _ w1017 w1073 _ _ _ _ _ _ _ _ _ _ _ _ _ _ _ _ _ _ _ _ _ _ _ _ _ _ _ _ _]
              tunnel: w811 -> [_ _ _ w853 _ _ _ _ _ _ _ _ _ _ _ _ _ _ _ _ _ _ _ _ _ _ _ _ _ w1207 _ _ _ _ _ _ _ _ _ _ _ _ _]
              frame "cContourAct" {
                n305 = Select(t="1", s="cContourAct", f="0") -> (s? t:f=w820:string)
              }
              frame "cdColorbarLabel" {
                n306 = local read "mSingleColorbar Actual"() -> (w824:bool)
                n307 = local read "Plot Titles"() -> (w830:string[])
                n308 = global read "Results_plotter_Global.vi" "Legend of ch names"() -> (w832:string[])
                n309 = case shown="True" w824 {
                  tunnel: w832 -> [w838 w840]
                  tunnel: w825 -> [w837 _]
                  tunnel: [w836 w841] -> w827
                  frame False {
                    n310 = Index Array(array=w838, index=w837) -> (element=w836:string)
                  }
                  frame True {
                    n311 = call "Analyse_string_array.vi"("String array"=w840) -> ("Unique strings"=w839:string[])  [unwired: 1 in, 1 out]
                    n312 = for {
                      shift-right: [w847] -> w843
                      shift-left: "" -> [w848]
                      tunnel: w839 -> [w846] mode=indexing
                      n313 = call <vilib>:"Space Constant.vi"() -> ("String"=w845:string)
                      n314 = Concatenate Strings(w848, w845, w846) -> (w847:string)
                    }
                    n315 = String Subset(string=w843, offset (0)=1) -> (substring=w841:string)  [unwired: 1 in]
                  }
                }
                n316 = Index Array(array=w830, index=w829) -> (element=w828:string)
                n317 = Equal?(x=w827, y=w828) -> (x = y?=w826:bool)
                n318 = case shown="False" w826 {
                  tunnel: [w834 ""] -> w831
                  tunnel: w827 -> [w833 _]
                  frame False {
                    n319 = call "TypesetInsideMathmode.vi"("DirtyString"=w833) -> ("Mathmode String"=w834:string)  [unwired: 8 in, 2 out]
                  }
                  frame True {
                  }
                }
              }
              frame "cdColorbarLogarithmic" {
                n320 = case shown="\"Lin\"" "Plotting" {
                  tunnel: ["0" ("fAxisLimY Location") "1" ("fAxisLimY Location")] -> w849
                  frame "Lin" {
                  }
                  frame "Log" {
                  }
                }
              }
              frame "cdColorbarRange" {
                n321 = local read "mSingleColorbar"() -> (w859:bool)
                n322 = local read "C limits"() -> (w865:dbl[][])
                n323 = case shown="True" w859 {
                  tunnel: w865 -> [w889 w895]
                  tunnel: [w887 w894] -> w860
                  tunnel: w858 -> [w888 w891]
                  tunnel: w853 -> [_ w890]
                  frame False {
                    n324 = Index Array(array=w889, index (row)=w888) -> (element=w887:dbl[])  [unwired: 1 in]
                  }
                  frame True {
                    n325 = global read "Results_plotter_Global.vi" "Ordinate Strings"() -> (w893:string[])
                    n326 = Array Size(array=w893) -> (size(s)=w892:i32)
                    n327 = case shown="1" w892 {
                      tunnel: w895 -> [w898 w907]
                      tunnel: [w897 w905] -> w894
                      tunnel: w891 -> [_ w910]
                      tunnel: w890 -> [w896 _]
                      frame 1 {
                        n328 = case shown="\"Mass Mode\"" w896 {
                          tunnel: w898 -> [_ w903]
                          tunnel: [w899 w902] -> w897
                          frame "Mass Mode" {
                            n329 = global read "Results_plotter_Global.vi" "Max plotted value"() -> (w900:dbl)
                            n330 = global read "Results_plotter_Global.vi" "Min plotted value"() -> (w901:dbl)
                            n331 = Build Array(w900, w901) -> (w899:dbl[])
                          }
                          frame Default {
                            n332 = for {
                              tunnel: [w904] -> w902 mode=concatenating
                              tunnel: w903 -> [w904] mode=indexing
                            }
                          }
                        }
                      }
                      frame 2, Default {
                        n333 = local read "Ord strngs"() -> (w909:string[])
                        n334 = Index Array(array=w909, index=w910) -> (element=w908:string)
                        n335 = for {
                          tunnel: w909 -> [w916] mode=indexing
                          tunnel: w908 -> [w915]
                          shift-right: [w911] -> w905
                          shift-left: dbl[] [] -> [w913]
                          tunnel: w907 -> [w912] mode=indexing
                          n336 = Equal?(x=w916, y=w915) -> (x = y?=w914:bool)
                          n337 = case shown="True" w914 {
                            tunnel: w913 -> [w917 w920]
                            tunnel: w912 -> [_ w919]
                            tunnel: [w917 w918] -> w911
                            frame False {
                            }
                            frame True {
                              n338 = Build Array (concatenate)(w920, w919) -> (w918:dbl[])
                            }
                          }
                        }
                      }
                    }
                  }
                }
                n339 = local read "Concentration?"() -> (w854:bool)
                n340 = case shown="False" w854 {
                  tunnel: [w870 w876] -> w862
                  tunnel: [w866 w875] -> w861
                  tunnel: w860 -> [w873 w874]
                  frame False {
                    n341 = Array Max & Min(array=w873) -> (max value=w868:dbl, min value=w869:dbl)  [unwired: 2 out]
                    n342 = Subtract(x=w868, y=w869) -> (x-y=w872:dbl)
                    n343 = Multiply(x=0.05, y=w872) -> (x*y=w867:dbl)
                    n344 = Subtract(x=w869, y=w867) -> (x-y=w870:dbl)
                    n345 = Add(x=w868, y=w867) -> (x+y=w866:dbl)
                  }
                  frame True {
                    n346 = call <vilib>:"Std Deviation and Variance.vi"("X"=w874) -> ("mean"=w878:dbl, "standard deviation"=w879:dbl)  [unwired: 1 in, 1 out]
                    n347 = Multiply(x=w879, y=4.0) -> (x*y=w881:dbl)
                    n348 = Multiply(x=w879, y=6.0) -> (x*y=w877:dbl)
                    n349 = Subtract(x=w878, y=w877) -> (x-y=w876:dbl)
                    n350 = Add(x=w878, y=w881) -> (x+y=w875:dbl)
                  }
                }
                n351 = local read "Plotting"() -> (w864:enum8{"Lin", "Log"})
                n352 = case shown="\"Log\"" w864 {
                  tunnel: [w921 w924] -> w863
                  tunnel: w862 -> [w921 w922]
                  tunnel: w861 -> [_ w927]
                  tunnel: "No Of decades" -> [_ w926]
                  frame "Lin" {
                  }
                  frame "Log" {
                    n353 = case shown="6" w926 {
                      tunnel: [100.0 1000.0 10000.0 100000.0 1000000.0 10000000.0 10.0] -> w925
                      frame 2 {
                      }
                      frame 3 {
                      }
                      frame 4 {
                      }
                      frame 5 {
                      }
                      frame 6 {
                      }
                      frame 7, Default {
                      }
                      frame 1 {
                      }
                    }
                    n354 = Divide(x=w927, y=w925) -> (x/y=w923:dbl)
                    n355 = Max & Min(x=w922, y=w923) -> (max(x,y)=w924:dbl)  [unwired: 1 out]
                  }
                }
                n356 = case shown="True" "Range Auto" {
                  tunnel: w863 -> [_ w885]
                  tunnel: w861 -> [_ w886]
                  tunnel: ["cdColorbarRange" w884] -> w855
                  frame False {
                  }
                  frame True {
                    n357 = call "Non equal Min Max.vi"("Max"=w886, "Min"=w885) -> ("Limits"=w884:string)  [unwired: 1 in]
                    n358 = local write "cdColorbarRange"(w884) -> ()
                  }
                }
              }
              frame "cdMethodInterp" {
                n359 = local read "Plotting"() -> (w935:enum8{"Lin", "Log"})
                n360 = case shown="\"Log\"" w935 {
                  tunnel: ["cubic" "natural"] -> w936
                  frame "Lin" {
                  }
                  frame "Log" {
                  }
                }
              }
              frame "cdSpaceInterp" {
                n361 = case shown="-1" w941 {
                  tunnel: w943 -> [_ w952]
                  tunnel: [w944 w947] -> w942
                  tunnel: w940 -> [w946 _]
                  tunnel: w939 -> [w945 _]
                  frame -1 {
                    n362 = Index Array(array=w946, index=w945) -> (element=w944:string)
                  }
                  frame Default {
                    n363 = local read "Max dimension per figure"() -> (w953:dbl[])
                    n364 = Index Array(array=w953, index=w952) -> (element=w951:dbl)
                    n365 = Divide(x=w951, y=300.0) -> (x/y=w948:dbl)
                    n366 = Format Into String(format string="%.0e", w948) -> (resulting string=w947:string)  [unwired: 2 in, 1 out]
                  }
                }
              }
              frame "cLevNr" {
                n367 = Number To Decimal String(number="Number of Contours") -> (decimal integer string=w955:string)  [unwired: 1 in]
              }
              frame "cLineStyle" {
                n368 = local read "Streamlines"() -> (w956:bool)
                n369 = Select(t="none", s=w956, f="-") -> (s? t:f=w957:string)
              }
              frame "cScatterAct" {
                n370 = Select(t="1", s="cScatterAct", f="0") -> (s? t:f=w960:string)
              }
              frame "cScatterPointSize" {
                n371 = local read "Number of Figures"() -> (w967:i32)
                n372 = Fract/Exp String To Number(string="cScatterPointSize") -> (number=w968:dbl)  [unwired: 3 in, 1 out]
                n373 = Divide(x=w968, y=w967) -> (x/y=w966:dbl)
                n374 = Number To Fractional String(number=w966, precision (6)=i16 2) -> (F-format string=w964:string)  [unwired: 2 in]
              }
              frame "fAxisLabelX" {
                n375 = local read "Plot X Axis"() -> (w971:i32[])
                n376 = Index Array(array=w971, index=w974) -> (element=w985:i32)
                n377 = Array Max & Min(array=w971) -> (max value=w973:i32, min value=w972:i32)  [unwired: 2 out]
                n378 = Equal?(x=w973, y=w972) -> (x = y?=w970:bool)
                n379 = case shown="False" w970 {
                  tunnel: [TRUE w991] -> w977
                  tunnel: w974 -> [_ w990]
                  frame False {
                  }
                  frame True {
                    n380 = local read "X Labels"() -> (w992:bool[])
                    n381 = Index Array(array=w992, index=w990) -> (element=w991:bool)
                  }
                }
                n382 = global read "Results_plotter_Global.vi" "3D Ch Names"() -> (w986:string[])
                n383 = Index Array(array=w986, index=w985) -> (element=w978:string)
                n384 = call "Fast_string_Replace.vi"("Replace match with:"=" ", "Input String"=w978, "matchThis"=":" ("regular expression")) -> ("Output String"=w982:string)  [unwired: 1 in, 1 out]
                n385 = call "Fast_string_Replace.vi"("Replace match with:"=" ", "Input String"=w982, "matchThis"="  " ("regular expression")) -> ("Output String"=w981:string)  [unwired: 1 in, 1 out]
                n386 = call <vilib>:"Trim Whitespace.vi"("string"=w981) -> ("trimmed string"=w976:string)  [unwired: 1 in]
                n387 = call "TypesetInsideMathmode.vi"("DirtyString"=w976) -> ("Mathmode String"=w975:string)  [unwired: 8 in, 2 out]
                n388 = Select(t=w975, s=w977, f="") -> (s? t:f=w987:string)
              }
              frame "fAxisLabelY" {
                n389 = local read "Plot Y Axis"() -> (w996:i32[])
                n390 = Index Array(array=w996, index=w997) -> (element=w1007:i32)
                n391 = Array Max & Min(array=w996) -> (max value=w995:i32, min value=w994:i32)  [unwired: 2 out]
                n392 = Equal?(x=w995, y=w994) -> (x = y?=w993:bool)
                n393 = case shown="False" w993 {
                  tunnel: [TRUE w1014] -> w1008
                  tunnel: w997 -> [_ w1013]
                  frame False {
                  }
                  frame True {
                    n394 = local read "Y labels"() -> (w1015:bool[])
                    n395 = Index Array(array=w1015, index=w1013) -> (element=w1014:bool)
                  }
                }
                n396 = global read "Results_plotter_Global.vi" "3D Ch Names"() -> (w1009:string[])
                n397 = Index Array(array=w1009, index=w1007) -> (element=w1000:string)
                n398 = call "Fast_string_Replace.vi"("Replace match with:"=" ", "Input String"=w1000, "matchThis"=":" ("regular expression")) -> ("Output String"=w1004:string)  [unwired: 1 in, 1 out]
                n399 = call "Fast_string_Replace.vi"("Replace match with:"=" ", "Input String"=w1004, "matchThis"="  " ("regular expression")) -> ("Output String"=w1003:string)  [unwired: 1 in, 1 out]
                n400 = call <vilib>:"Trim Whitespace.vi"("string"=w1003) -> ("trimmed string"=w999:string)  [unwired: 1 in]
                n401 = call "TypesetInsideMathmode.vi"("DirtyString"=w999) -> ("Mathmode String"=w998:string)  [unwired: 8 in, 2 out]
                n402 = Select(t=w998, s=w1008, f="") -> (s? t:f=w1010:string)
              }
              frame "fAxisLimX" {
                n403 = case shown="-1" w1019 {
                  tunnel: w1020 -> [w1023 _]
                  tunnel: w1018 -> [_ w1071]
                  tunnel: w1017 -> [_ w1070]
                  tunnel: [w1021 w1069] -> w1016
                  frame Default {
                    n404 = case shown="True" "X Limits Auto" {
                      tunnel: ["Location X limits" w1026] -> w1021
                      tunnel: w1023 -> [_ w1030]
                      tunnel: "Show Source" -> [_ w1029]
                      frame False {
                      }
                      frame True {
                        n405 = local read "Source locations"() -> (w1031:string[])
                        n406 = local read "Plot X Axis"() -> (w1034:i32[])
                        n407 = Index Array(array=w1034, index=w1030) -> (element=w1033:i32)
                        n408 = case shown="True" "Same Location limits for all plots" {
                          tunnel: [w1040 w1056] -> w1028
                          tunnel: [w1039 w1055] -> w1027
                          tunnel: w1033 -> [w1042 w1053]
                          tunnel: w1030 -> [w1048 _]
                          tunnel: w1031 -> [w1046 w1054]
                          tunnel: w1030 -> [w1045 _]
                          tunnel: w1029 -> [w1037 w1052]
                          frame False {
                            n409 = Index Array(array=w1046, index=w1045) -> (element=w1044:string)
                            n410 = local read "Limits Array"() -> (w1047:dbl[][][])
                            n411 = call "Get_array_values_fr_String.vi"("String Value"=w1044) -> ("Numeric Array"=w1043:dbl[])  [unwired: 1 out]
                            n412 = Index Array(array=w1043, index=w1042) -> (element=w1041:dbl)
                            n413 = Index Array(array=w1047, index (dim 0)=w1048) -> (element=w1049:dbl[][])  [unwired: 2 in]
                            n414 = Index Array(array=w1049, index (row)=w1042) -> (element=w1036:dbl[])  [unwired: 1 in]
                            n415 = Build Array (concatenate)(w1036, w1041) -> (w1038:dbl[])
                            n416 = Select(t=w1038, s=w1037, f=w1036) -> (s? t:f=w1035:dbl[])
                            n417 = Array Max & Min(array=w1035) -> (max value=w1040:dbl, min value=w1039:dbl)  [unwired: 2 out]
                          }
                          frame True {
                            n418 = case shown="0, Default" w1053 {
                              tunnel: [w1066 w1067 w1068] -> w1051
                              frame 0, Default {
                                n419 = local read "All X"() -> (w1066:dbl[])
                              }
                              frame 1 {
                                n420 = local read "All Y"() -> (w1067:dbl[])
                              }
                              frame 2 {
                                n421 = local read "All Z"() -> (w1068:dbl[])
                              }
                            }
                            n422 = case shown="False" w1052 {
                              tunnel: w1054 -> [_ w1063]
                              tunnel: w1053 -> [_ w1061]
                              tunnel: w1051 -> [w1057 w1059]
                              tunnel: [w1057 w1058] -> w1050
                              frame False {
                              }
                              frame True {
                                n423 = for {
                                tunnel: w1063 -> [w1065] mode=indexing
                                tunnel: [w1064] -> w1062 mode=indexing
                                n424 = call "Get_array_values_fr_String.vi"("String Value"=w1065) -> ("Numeric Array"=w1064:dbl[])  [unwired: 1 out]
                                }
                                n425 = Index Array(array=w1062, index (col)=w1061) -> (element=w1060:dbl[])  [unwired: 1 in]
                                n426 = Build Array (concatenate)(w1060, w1059) -> (w1058:dbl[])
                              }
                            }
                            n427 = Array Max & Min(array=w1050) -> (max value=w1056:dbl, min value=w1055:dbl)  [unwired: 2 out]
                          }
                        }
                        n428 = call "Set Plot limits.vi"("Min"=w1027, "Max"=w1028) -> ("resulting string"=w1026:string)
                      }
                    }
                  }
                  frame -1 {
                    n429 = Index Array(array=w1071, index=w1070) -> (element=w1069:string)
                  }
                }
                "X Limit" <- w1016
              }
              frame "fAxisLimY" {
                n430 = case shown="-1" w1074 {
                  tunnel: w1076 -> [w1078 _]
                  tunnel: [w1077 w1102] -> w1075
                  tunnel: w1073 -> [_ w1104]
                  tunnel: w1072 -> [_ w1103]
                  frame Default {
                    n431 = case shown="True" "Y Limits Auto" {
                      tunnel: ["Location Y limits" w1081] -> w1077
                      tunnel: w1078 -> [_ w1084]
                      frame False {
                      }
                      frame True {
                        n432 = local read "Plot Y Axis"() -> (w1087:i32[])
                        n433 = local read "Same Location limits for all plots"() -> (w1085:bool)
                        n434 = Index Array(array=w1087, index=w1084) -> (element=w1086:i32)
                        n435 = case shown="False" w1085 {
                          tunnel: [w1093 w1096] -> w1083
                          tunnel: [w1092 w1095] -> w1082
                          tunnel: w1086 -> [w1090 w1098]
                          tunnel: w1084 -> [w1089 _]
                          frame False {
                            n436 = local read "Limits Array"() -> (w1088:dbl[][][])
                            n437 = Index Array(array=w1088, index (dim 0)=w1089) -> (element=w1091:dbl[][])  [unwired: 2 in]
                            n438 = Index Array(array=w1091, index (row)=w1090) -> (element=w1094:dbl[])  [unwired: 1 in]
                            n439 = Index Array(array=w1094) -> (element #1=w1093:dbl, element #2=w1092:dbl)  [unwired: 2 in]
                          }
                          frame True {
                            n440 = case shown="2" w1098 {
                              tunnel: [w1099 w1100 w1101] -> w1097
                              frame 0, Default {
                                n441 = local read "All X"() -> (w1099:dbl[])
                              }
                              frame 1 {
                                n442 = local read "All Y"() -> (w1100:dbl[])
                              }
                              frame 2 {
                                n443 = local read "All Z"() -> (w1101:dbl[])
                              }
                            }
                            n444 = Array Max & Min(array=w1097) -> (max value=w1096:dbl, min value=w1095:dbl)  [unwired: 2 out]
                          }
                        }
                        n445 = call "Set Plot limits.vi"("Min"=w1082, "Max"=w1083) -> ("resulting string"=w1081:string)
                      }
                    }
                  }
                  frame -1 {
                    n446 = Index Array(array=w1103, index=w1104) -> (element=w1102:string)
                  }
                }
                "Y Limit" <- w1075
              }
              frame "fFigureNr" {
                n447 = Increment(x=w1107) -> (x+1=w1105:i32)
                n448 = Number To Decimal String(number=w1105) -> (decimal integer string=w1106:string)  [unwired: 1 in]
              }
              frame "fFlipNormal" {
                n449 = local read "Plot X Axis"() -> (w1114:i32[])
                n450 = local read "Plot Y Axis"() -> (w1112:i32[])
                n451 = Index Array(array=w1114, index=w1111) -> (element=w1113:i32)
                n452 = Index Array(array=w1112, index=w1111) -> (element=w1110:i32)
                n453 = case shown="0" w1113 {
                  tunnel: w1110 -> [w1117 _]
                  tunnel: [w1116 w1120] -> w1109
                  tunnel: "0;0" -> [w1115 w1120]
                  frame 0 {
                    n454 = case shown="Default" w1117 {
                      tunnel: [w1118 "2;2"] -> w1116
                      tunnel: w1115 -> [w1118 _]
                      frame Default {
                      }
                      frame 2 {
                      }
                    }
                  }
                  frame Default {
                  }
                }
              }
              frame "fReverseAxis" {
                n455 = local read "Constant Axis"() -> (w1124:i32[])
                n456 = Index Array(array=w1124, index=w1123) -> (element=w1122:i32)
                n457 = case shown="1" w1122 {
                  tunnel: ["0;1" "0;0" "0;0"] -> w1121
                  frame 0, Default {
                  }
                  frame 1 {
                  }
                  frame 2 {
                  }
                }
              }
              frame "fShowFigure" {
                n458 = Select(t="1", s="Interactive Window", f="0") -> (s? t:f=w1128:string)
              }
              frame "fTickLabel" {
                n459 = local read "Show all Axis"() -> (w1132:bool)
                n460 = case shown="False" w1132 {
                  tunnel: [w1136 FALSE ("Same Location limits for all plots")] -> w1133
                  frame False {
                    n461 = local read "Same Location limits for all plots"() -> (w1136:bool)
                  }
                  frame True {
                  }
                }
                n462 = case shown="True" w1133 {
                  tunnel: ["1;1" w1146] -> w1135
                  tunnel: w1134 -> [_ w1139]
                  frame False {
                  }
                  frame True {
                    n463 = local read "nRows"() -> (w1145:u8)
                    n464 = local read "nCols"() -> (w1143:u8)
                    n465 = local read "X Labels"() -> (w1156:bool[])
                    n466 = local read "Y labels"() -> (w1150:bool[])
                    n467 = Increment(x=w1145) -> (x+1=w1144:u8)
                    n468 = Index Array(array=w1156, index=w1139) -> (element=w1141:bool)
                    n469 = Greater?(x=w1143, y=w1144) -> (0:w1142:bool)
                    n470 = Index Array(array=w1150, index=w1139) -> (element=w1151:bool)
                    n471 = Or(x=w1142, y=w1141) -> (x .or. y?=w1140:bool)
                    n472 = Select(t="1", s=w1151, f="0") -> (s? t:f=w1149:string)
                    n473 = Select(t="1", s=w1140, f="0") -> (s? t:f=w1148:string)
                    n474 = Concatenate Strings(w1148, ";" ("string"), w1149) -> (w1146:string)
                  }
                }
              }
              frame "fTitle" {
                n475 = local read "Plot Titles"() -> (w1160:string[])
                n476 = local read "Math titles"() -> (w1158:bool)
                n477 = Index Array(array=w1160, index=w1161) -> (element=w1159:string)
                n478 = case shown="False" w1158 {
                  tunnel: w1159 -> [w1162 w1164]
                  tunnel: [w1162 w1163] -> w1157
                  frame False {
                  }
                  frame True {
                    n479 = call "TypesetInsideMathmode.vi"("DirtyString"=w1164) -> ("Mathmode String"=w1163:string)  [unwired: 8 in, 2 out]
                  }
                }
              }
              frame "fVectorComponentNr" {
                n480 = local read "Streamlines"() -> (w1167:bool)
                n481 = local read "Vectors"() -> (w1166:bool)
                n482 = Or(x=w1166, y=w1167) -> (x .or. y?=w1165:bool)
                n483 = Select(t="3", s=w1165, f="0") -> (s? t:f=w1168:string)
              }
              frame "fVectorRotations" {
              }
              frame "gGeometryAct" {
                n484 = local read "stl file"() -> (w1173:string)
                n485 = Empty String/Path?(string/path=w1173) -> (empty?=w1172:bool)
                n486 = Select(t="0", s=w1172, f="1") -> (s? t:f=w1176:string)
              }
              frame "gldGeometryFilename" {
                n487 = local read "stl file"() -> (w1177:string)
              }
              frame "gldGeometryRotations" {
                n488 = case shown="True" "Rotate Model?" {
                  tunnel: ["0;0;0" ("format string") w1185] -> w1180
                  tunnel: w1178 -> [_ w1184]
                  frame False {
                  }
                  frame True {
                    n489 = local read "Wind Directions"() -> (w1183:dbl[])
                    n490 = Index Array(array=w1183, index=w1184) -> (element=w1182:dbl)
                    n491 = Negate(x=w1182) -> (-x=w1186:dbl)
                    n492 = Format Into String(format string="0;0;%.0f", w1186) -> (resulting string=w1185:string)  [unwired: 2 in, 1 out]
                  }
                }
              }
              frame "ldRefPointColor" {
                n493 = local read "Show Source"() -> (w1191:bool)
                n494 = Select(t="Source Color", s=w1191, f="") -> (s? t:f=w1188:string)
              }
              frame "ldRefPointCoord" {
                n495 = local read "Source locations"() -> (w1197:string[])
                n496 = Index Array(array=w1197, index=w1196) -> (element=w1193:string)
                n497 = local read "Show Source"() -> (w1195:bool)
                n498 = Select(t=w1193, s=w1195, f="") -> (s? t:f=w1192:string)
              }
              frame "ldRefPointSize" {
                n499 = local read "Show Source"() -> (w1201:bool)
                n500 = Select(t="Source Size", s=w1201, f="") -> (s? t:f=w1199:string)
              }
              frame "ldViewAngles" {
                n501 = Select(t="90;90", s="Flip vertical and Horizontal axes", f="0;90") -> (s? t:f=w1203:string)
              }
              frame "mFormatFig" {
                n502 = case shown="Default" w1207 {
                  tunnel: ["pdf" "png"] -> w1206
                  frame Default {
                  }
                  frame "Mass Mode" {
                  }
                }
                "Output format" <- w1206
              }
              frame "mGraphsxColumn" {
                n503 = Number To Decimal String(number="nCols") -> (decimal integer string=w1210:string)  [unwired: 1 in]
              }
              frame "mGraphsxRow" {
                n504 = Number To Decimal String(number="nRows") -> (decimal integer string=w1212:string)  [unwired: 1 in]
              }
              frame "mMainTitle" {
                n505 = local read "Final Title"() -> (w1215:string)
                n506 = call "TypesetInsideMathmode.vi"("DirtyString"=w1215) -> ("Mathmode String"=w1214:string)  [unwired: 8 in, 2 out]
              }
              frame "mMainTitleFontSize" {
              }
              frame "mFontSize" {
              }
              frame "mSingleColorbar" {
                n507 = local read "mSingleColorbar Actual"() -> (w1218:bool)
                n508 = Select(t="1", s=w1218, f="0") -> (s? t:f=w1219:string)
              }
              frame "mSingleColorbarLocation" {
                n509 = Format Into String(format string="%s;%s;%s;%s", "LeftEdge", "BottomEdge", "Width", "Height") -> (resulting string=w1222:string)  [unwired: 2 in, 1 out]
              }
              frame "mSpaceX" {
                n510 = local read "Same Location limits for all plots"() -> (w1229:bool)
                n511 = case shown="False" w1229 {
                  tunnel: ["2.2" ("f") w1232] -> w1228
                  frame False {
                  }
                  frame True {
                    n512 = local read "mSingleColorbar Actual"() -> (w1231:bool)
                    n513 = case shown="True" w1231 {
                      tunnel: ["0.4" "0.35"] -> w1232
                      frame False {
                      }
                      frame True {
                      }
                    }
                  }
                }
              }
              frame "mSpaceY" {
                n514 = local read "Show all Axis"() -> (w1236:bool)
                n515 = case shown="True" w1236 {
                  tunnel: [w1241 FALSE ("Same Location limits for all plots")] -> w1239
                  tunnel: ["1.6" ("f") "1.8" ("f")] -> w1235
                  frame False {
                    n516 = local read "Same Location limits for all plots"() -> (w1241:bool)
                  }
                  frame True {
                  }
                }
                n517 = Select(t="0.7", s=w1239, f=w1235) -> (s? t:f=w1237:string)
              }
              frame "mBottomEdge" {
                n518 = local read "mSingleColorbar Actual"() -> (w1244:bool)
                n519 = Select(t="3.2", s=w1244, f="1.5") -> (s? t:f=w1245:string)
              }
              frame "tStreamlineAct" {
                n520 = Select(t="1", s="Streamlines", f="0") -> (s? t:f=w1249:string)
              }
              frame "vVectorAct" {
                n521 = Select(t="1", s="Vectors", f="0") -> (s? t:f=w1253:string)
              }
              frame Default {
              }
            }
          }
        }
        n522 = Build Array (concatenate)(w794, w795) -> (→"Table":string[][])
      }
      frame "Save Input File" {
        # "Create matching output directory, as MATLAB won't, and it may not exist, if running from EXE"
        n523 = local read "Source Y Location"() -> (w1266:u16)
        n524 = local read "Source Z Location"() -> (w1265:u16)
        n525 = local read "Source X Location"() -> (w1267:u16)
        n526 = local read "U Vector"() -> (w1271:u16)
        n527 = local read "W Vector"() -> (w1273:u16)
        n528 = local read "V Vector"() -> (w1272:u16)
        n529 = local read "Selectors"() -> (w1275:i32[])
        n530 = Build Array(w1271, w1272, w1273, w1267, w1266, w1265) -> (w1274:u16[])
        n531 = local read "Table"() -> (w1277:string[][])
        n532 = for {
          tunnel: w1274 -> [w1289] mode=indexing
          tunnel: w1275 -> [w1287]
          tunnel: w1270 -> [w1292]
          tunnel: w1268 -> [w1290]
          tunnel: [w1289] -> w1276 mode=indexing
          tunnel: w1269 -> [w1288] mode=indexing
          i -> [w1286]
          n533 = Index Array(array=w1287, index=w1286) -> (element=w1285:i32)
          n534 = Equal?(x=w1289, y=w1285) -> (x = y?=w1291:bool)
          n535 = case shown="False" w1291 {
            tunnel: w1292 -> [w1298 _]
            tunnel: w1289 -> [w1297 _]
            tunnel: w1290 -> [w1296 _]
            tunnel: w1288 -> [w1293 _]
            frame False {
              n536 = Index Array(array=w1296, index=w1297) -> (element=w1295:string)
              n537 = call "Read_Write_Template.vi"("Template File"=w1298, "Mode"=Global_mode."Write Global to File", "Single Value In"=w1295, "Data type"=w1293) -> ()  [unwired: 4 in, 8 out]
            }
            frame True {
            }
          }
        }
        n538 = Build Path(base path=w1280, name or relative path="Input2D.xls") -> (appended path=w1281:path)
        n539 = Array To Spreadsheet String(array=w1277, 3:"%s" ("format string")) -> (spreadsheet string=w1282:string)  [unwired: 1 in]
        n540 = Write to Text File(file (use dialog)=w1281, text=w1282) -> (refnum out=w1263:refnum<file>, error out=w1264:errorcluster)  [unwired: 2 in, 1 out]
        n541 = Build Path(base path=w1260, name or relative path="Output") -> (appended path=w1262:path)
        n542 = Close File(refnum=w1263, error in=w1264) -> (error out=w1257:errorcluster)  [unwired: 1 out]
        n543 = Build Path(base path=w1262, name or relative path=w1259) -> (appended path=w1258:path)
        n544 = call <vilib>:"Create Directory Recursive.vi"("error in (no error)"=w1257, "directory"=w1258) -> ()  [unwired: 3 in, 3 out]
        n545 = local write "Selectors"(w1276) -> ()
      }
      frame "Run MATLAB Code" {
        n546 = call "Call_MATLAB_Suite.vi"("Mode"=MATLAB_Mode."2D Plotter") -> ("Output file"=w1305:path, "error out"=w1299:errorcluster)  [unwired: 2 in, 1 out]
        "Output file" <- w1305
        n547 = case shown="Default" w1306 {
          tunnel: [FALSE ("Top Level") w1321] -> w1307
          tunnel: w1305 -> [w1315 w1320]
          tunnel: [w1314 w1320] -> w1304
          tunnel: w1299 -> [_ w1319]
          frame "Mass Mode" {
            n548 = Strip Path(path=w1315) -> (stripped path=w1309:path, name=w1316:string)
            n549 = local read "Output format"() -> (w1311:string)
            n550 = call "Add_filename_suffix.vi"("Filename"=w1316) -> ("Base name"=w1313:string)  [unwired: 1 in, 3 out]
            n551 = Concatenate Strings(w1313, ".", w1311) -> (w1312:string)
            n552 = Build Path(base path=w1309, name or relative path=w1312) -> (appended path=w1314:path)
          }
          frame Default {
            n553 = case shown="No Error" w1319 {
              selector: w1319 -> [_ w1325]
              tunnel: [TRUE ("Top Level") FALSE ("Top Level")] -> w1321
              tunnel: ["" ("source") w1324] -> w1318
              frame No Error {
              }
              frame Error {
                n554 = Unbundle By Name(w1325) -> ("source"=w1324:string)
                n555 = One Button Dialog(message=w1324) -> ()  [unwired: 1 in, 1 out]
              }
            }
            "Error String" <- w1318
          }
        }
        "Plot data file" <- w1304
        n556 = Select(t="Display PDF with save option", s="Show Save Option?", f="Display PDF" ("t")) -> (s? t:f=w1300:string)
      }
      frame "Display PDF with save option" {
        n557 = local read "Output file"() -> (w1328:path)
        n558 = stacked-sequence {
          tunnel: w1328 -> [w1333 w1347]
          frame #0 {
            n559 = local read "Data Dir"() -> (w1330:string[])
            n560 = call "Display PDF File for Preview.vi"("Data Directories"=w1330, "PDF file"=w1333) -> ("Filename Out"=w1331:string)  [unwired: 8 in, 1 out]
            n561 = Empty String/Path?(string/path=w1331) -> (empty?=w1332:bool)
            n562 = case shown="False" w1332 {
              tunnel: w1333 -> [w1339 _]
              tunnel: w1331 -> [w1338 _]
              tunnel: w1330 -> [w1337 _]
              frame False {
                n563 = local read "Duplicate Plot"() -> (w1340:bool)
                n564 = call "Save PDF files.vi"("Duplicate Plot"=w1340, "Open in Acrobat"="Open in Acrobat", "Desired Filename"=w1338, "Data Directories"=w1337, "PDF file in"=w1339) -> ("Results Folders"=w1334:path[])  [unwired: 5 in, 1 out]
                n565 = call "Save Plotted Data File Rows.vi"("Results Folders"=w1334) -> ()  [unwired: 5 in]
                n566 = global read "Results_plotter_Global.vi" "Template"() -> (w1336:path)
                n567 = Strip Path(path=w1336) -> (name=w1335:string)  [unwired: 1 out]
                n568 = for {
                  tunnel: w1334 -> [w1346] mode=indexing
                  tunnel: w1336 -> [w1345]
                  tunnel: w1335 -> [w1343]
                  n569 = Strip Path(path=w1346) -> (stripped path=w1344:path)  [unwired: 1 out]
                  n570 = Build Path(base path=w1344, name or relative path=w1343) -> (appended path=w1342:path)
                  n571 = Copy(10:w1342, 11:w1345) -> ()  [unwired: 3 in, 3 out]
                }
              }
              frame True {
              }
            }
          }
          frame #1 {
            n572 = Delete(path (use dialog)=w1347) -> ()  [unwired: 4 in, 3 out]
          }
        }
      }
      frame "Display PDF" {
        n573 = local read "Output file"() -> (w1348:path)
        n574 = call "Open PDF in desired reader.vi"("Path"=w1348) -> ()  [unwired: 2 in, 1 out]
      }
      frame "End" {
      }
    }
  }
  "AuditTrail" <- w27
  "Saved Automatically?" <- FALSE
